vi "CRYAcquisition.vi"(0 "Setup in":T2={"No.VI"=0, "Category"="", "StepName"="", "Seq setup flattened"="", "Comment"="", "Steps config."=[], "Jump config"=[], "Start"=0.0, "Increment"=0.0, "Name"="Pa", "Unit"="Pa", "Y data"=1, "Y prefix"="", "Y dB ref"=1.0, "Y unit"="", "Repeat State Array"=[]} {"Repeat State Array"."Start" format="%#_5g"; "Y dB ref" format="%.1f"; "Y data" items=["dB", "Lin"]; "Start" format="%#_5g"}, 5 "Data In":T1[](array[typedef]) {"Z data" items=["dB", "Lin"]; "X data" items=["dB", "Lin"]; "Y data" items=["dB", "Lin"]; "Z dB ref" format="%.1f"; "Z axis" items=["Log", "Lin"]; "X dB ref" format="%.1f"; "X axis" items=["Log", "Lin"]; "Y axis" items=["Log", "Lin"]; "Y dB ref" format="%.1f"; "Curve"."z" format="%.2f"; "Curve"."y" format="%.2f"; "Curve"."x" format="%.2f"}, 7 "Results In":T4 {"Margin" format="%.2f"}, 9 "Seq Setup in":string, 11 "Step name":string="Play & Record", 12 "Hardware in":string, 13 "Calibration in":string) -> (3 "Types Out":string[](array[string]), 4 "Inserted Names Out":string[](array[string]), 6 "Data out":T1[](array[typedef]) {"Z data" items=["dB", "Lin"]; "X data" items=["dB", "Lin"]; "Y data" items=["dB", "Lin"]; "Z dB ref" format="%.1f"; "Z axis" items=["Log", "Lin"]; "X dB ref" format="%.1f"; "X axis" items=["Log", "Lin"]; "Y axis" items=["Log", "Lin"]; "Y dB ref" format="%.1f"; "Curve"."z" format="%.2f"; "Curve"."y" format="%.2f"; "Curve"."x" format="%.2f"}, 8 "Results out":T4 {"Margin" format="%.2f"}, 10 "Wave out":T3[](array[typedef]) {"Y dB ref" format="%.1f"; "Y axis" items=["Log", "Lin"]; "Y data" items=["dB", "Lin"]; "X data" items=["dB", "Lin"]})   [LabVIEW 2013]
doc: "This VI uses the Windows '95 multimedia system to play an audio waveform stream, and simultaneously record an input stream."
uses:
  Typedef Control/CRYResult Cluster Array.ctl
  Typedef Control/CRYResult Cluster.ctl
  Typedef Control/CRYData Cluster.ctl
  Typedef Control/CRYWaveform Cluster.ctl
  Typedef Control/CRYStep.ctl
  CRYMainGlobal.vi
  Misc/CRYOptions.vi
  Misc/SubVI/CRYMisc vis settings global.vi
  Calibration/SubVI/CRYCal Global.vi
  Task Sequence/CRYProject Run Control Global.vi
  CRYSound.dll
  Hardware/SubVI/CRY6175APT_Win32.dll
panel:
  in  "Record [ms]":dbl
  out "Acquisition Type":u16
  out "Index for testinfor":i32
  out "Numeric":i32
  in  "Datum":T1={"Name"="", "Curve"=[], "X data"=1, "Y data"=1, "Z data"=1, "X axis"=0, "Y axis"=1, "Z axis"=1, "X unit"="", "Y unit"="", "Z unit"="", "X dB ref"=1.0, "Y dB ref"=1.0, "Z dB ref"=1.0, "single val"=FALSE, "protected"=FALSE, "display X"=TRUE, "display Y"=FALSE, "display Z"=TRUE, "Test Info"="", "Step No."=0, "Plot Settings"={"Color"=0, "Interpolation"=0, "Point Style"=0, "Line Style"=0, "Point Color"=0, "Line Width"=0, "Bar Plot Style"=0, "Fill To"=0}, "AutoProtect"=FALSE} {"Z data" items=["dB", "Lin"]; "X data" items=["dB", "Lin"]; "Y data" items=["dB", "Lin"]; "Z dB ref" format="%.1f"; "Z axis" items=["Log", "Lin"]; "X dB ref" format="%.1f"; "X axis" items=["Log", "Lin"]; "Y axis" items=["Log", "Lin"]; "Y dB ref" format="%.1f"; "Curve"."z" format="%.2f"; "Curve"."y" format="%.2f"; "Curve"."x" format="%.2f"}
  out "Verdict":bool=TRUE
  out "Y dB ref":dbl
  in  "Waveform Cluster":T3={"Waveform"={"X0"=0.0, "dX"=0.0, "Y"=[]}, "X data"=1, "Y data"=1, "Y axis"=1, "X unit"="s", "Y unit"="V", "Y dB ref"=1.0, "display Y"=TRUE, "display X"=TRUE, "Overload?"=FALSE, "Test Info"="", "Step No."=0, "Name"="", "protected"=FALSE, "Sqc history"=[], "Signal Channel ID"=0, "Plot Settings"={"Color"=0, "Interpolation"=0, "Point Style"=0, "Line Style"=0, "Point Color"=0, "Line Width"=0, "Bar Plot Style"=0, "Fill To"=0}, "AutoProtect"=FALSE} {"Y dB ref" format="%.1f"; "Y axis" items=["Log", "Lin"]; "Y data" items=["dB", "Lin"]; "X data" items=["dB", "Lin"]}
  in  "ntaskID":u32
  in  "interact rec":bool
  in  "Record Delay":dbl caption="ms" format="%.1f"
  in  "interact play":bool
  in  "Max Out":dbl=3.0 format="%.3f"
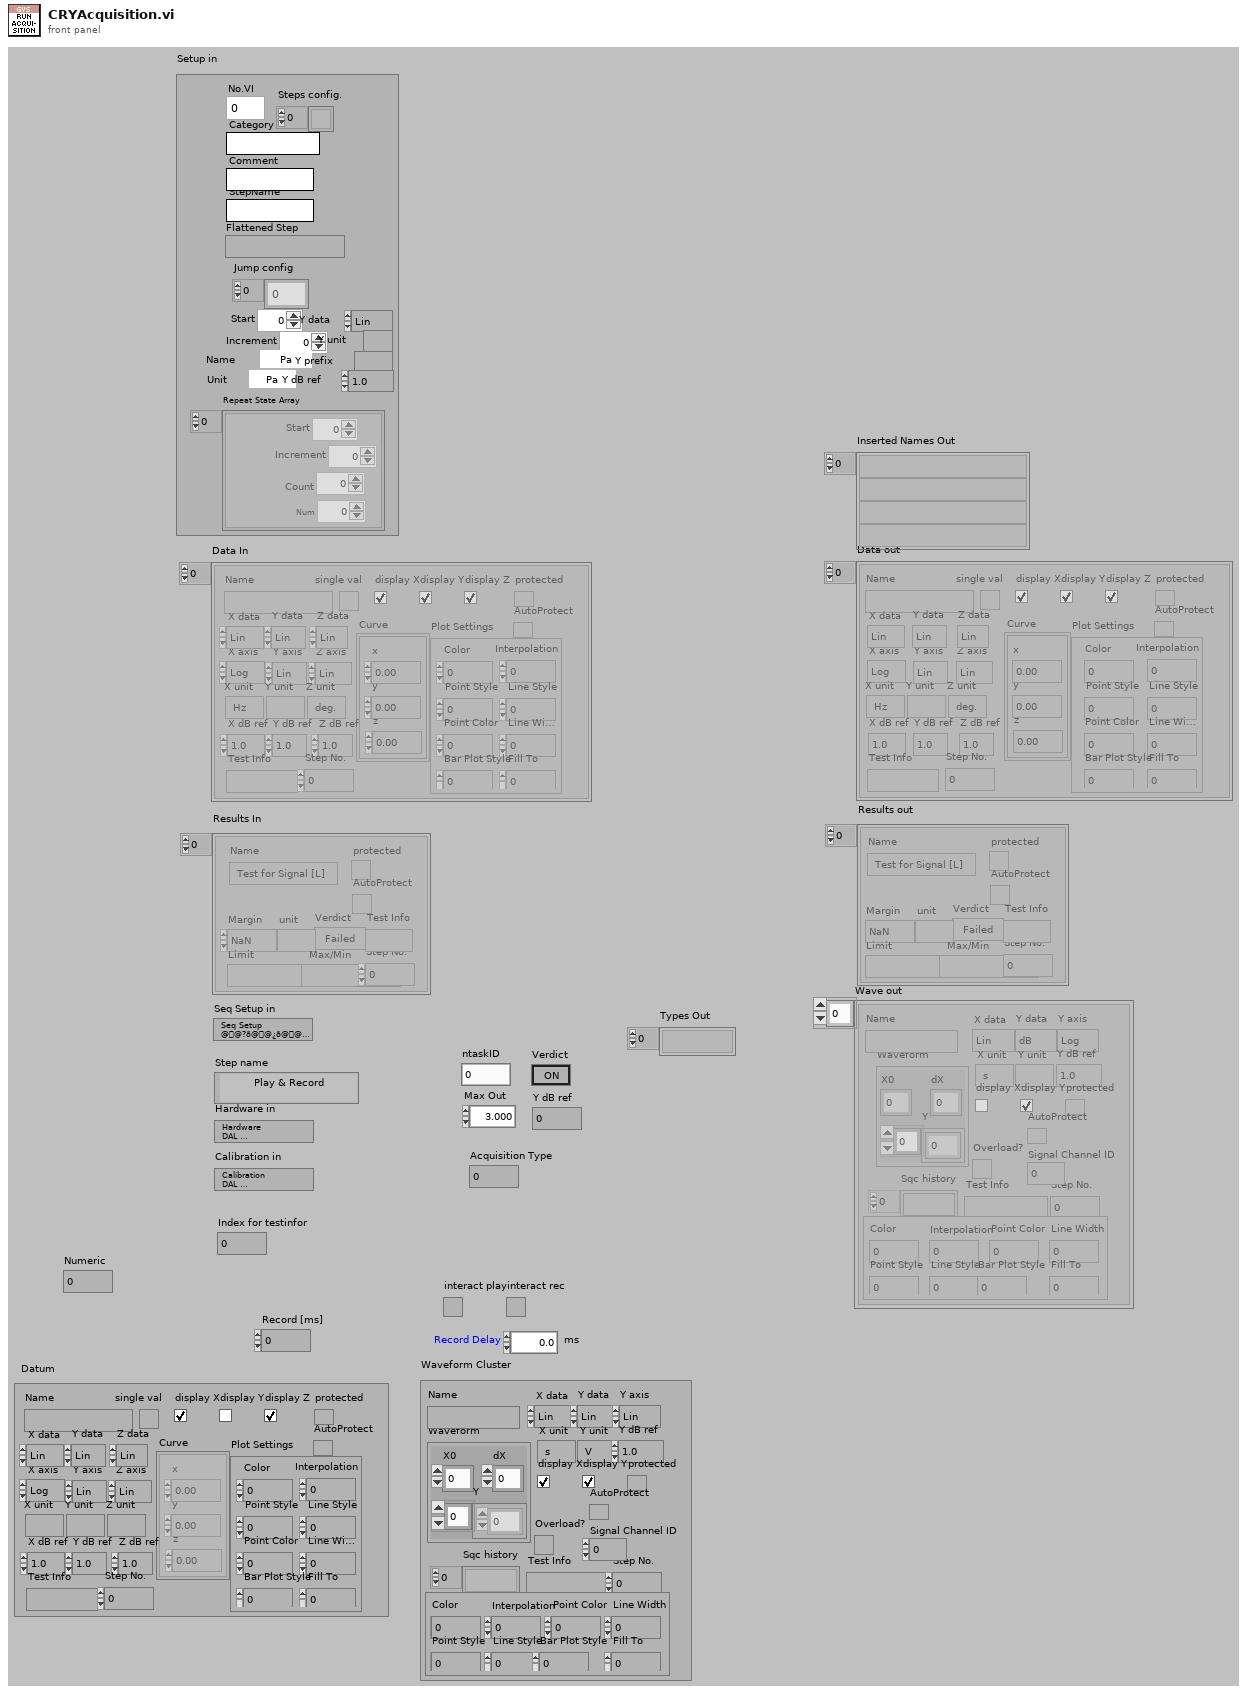
[diagram p1: front panel]
types:
  T1 = typedef "CRYData Cluster.ctl" = cluster{"Name":string, "Curve":cluster{"x":dbl, "y":dbl, "z":dbl}[], "X data":u16, "Y data":u16, "Z data":u16, "X axis":u16, "Y axis":u16, "Z axis":u16, "X unit":string, "Y unit":string, "Z unit":string, "X dB ref":dbl, "Y dB ref":dbl, "Z dB ref":dbl, "single val":bool, "protected":bool, "display X":bool, "display Y":bool, "display Z":bool, "Test Info":string, "Step No.":i32, "Plot Settings":cluster{"Color":u32, "Interpolation":u8, "Point Style":u8, "Line Style":u8, "Point Color":u32, "Line Width":u8, "Bar Plot Style":u8, "Fill To":i16}, "AutoProtect":bool}
  T2 = typedef "CRYStep.ctl" = cluster{"No.VI":i32, "Category":string, "StepName":string, "Seq setup flattened":string, "Comment":string, "Steps config.":bool[], "Jump config":i32[], "Start":dbl, "Increment":dbl, "Name":string, "Unit":string, "Y data":u16, "Y prefix":string, "Y dB ref":dbl, "Y unit":string, "Repeat State Array":cluster{"Start":dbl, "Increment":dbl, "Count":i32, "Num":i32}[]}
  T3 = typedef "CRYWaveform Cluster.ctl" = cluster{"Waveform":cluster{"X0":dbl, "dX":dbl, "Y":sgl[]}, "X data":u16, "Y data":u16, "Y axis":u16, "X unit":string, "Y unit":string, "Y dB ref":dbl, "display Y":bool, "display X":bool, "Overload?":bool, "Test Info":string, "Step No.":i32, "Name":string, "protected":bool, "Sqc history":string[], "Signal Channel ID":i32, "Plot Settings":cluster{"Color":u32, "Interpolation":u8, "Point Style":u8, "Line Style":u8, "Point Color":u32, "Line Width":u8, "Bar Plot Style":u8, "Fill To":i16}, "AutoProtect":bool}
  T4 = typedef "CRYResult Cluster Array.ctl" = T5[]
  T5 = typedef "CRYResult Cluster.ctl" = cluster{"Name":string, "Margin":dbl, "unit":string, "Verdict":bool, "Limit":string, "Max/Min":string, "protected":bool, "Step No.":i32, "Test Info":string, "AutoProtect":bool}
  T6 = enum16{"OK", "Yes", "YesNo", "YesNoCancel", "ReplaceAppend"}
  T7 = enum16{"Play & Record", "Record", "Sine Generator", "Voltmeter", "Oscilloscope", "Spectrum Analyzer", "RTA", "Generator & Voltmeter", "Generator & Oscilloscope", "Generator & Spectrum", "Generator & RTA"}
  T8 = typedef "CRYAcquisition Cluster.ctl" = cluster{"Mode":u16, "Name":string, "use ch name":bool, "Record Time":dbl, "hide rec":bool, "hide play":bool, "rec delay":dbl, "rec pad":dbl, "dcc units":i8, "sine gen setting":string, "scope_fft setting":string, "voltmeter setting":string, "rta setting":string, "trig offset(sec)":dbl, "triggered  record":bool, "trig level":dbl, "trig unit":u8, "trig slop":bool, "trig timeout(sec)":dbl, "add record":bool, "EQ":bool, "record table":string[][], "play table":string[][], "trig channel":string, "Help":string}
  T9 = typedef "CRYCalibration 2DCluster.ctl" = cluster{"Calibration":T10, "Corr Curve":T1, "EQ Curve":T1, "Sens Curve":T1}
  T10 = typedef "CRYCalibration Cluster.ctl" = cluster{"Calibration Step Name":string, "Device":string, "Correction Curve Name":string, "Equalization Curve Name":string, "Sensitivity Curve Name":string, "Corr Folder and File":string, "EQ Folder and File":string, "Sens Folder and File":string, "Corr Step size":u16, "EQ Step size":u16, "Input":bool, "Last Cal Date (sec)":timestamp, "Cha Name":string, "Corr Curve Found":bool, "EQ Curve Found":bool, "Sens Curve Found":bool, "Signal Type":string, "Calibrated Device":string, "Hz":u32}
  T11 = typedef "CRYCalibration All Cluster.ctl" = cluster{"Calibration 2D":T9[], "Help":string, "Tab Value":i32, "Input Signal Type":string, "Output Signal Type":string}
  T12 = typedef "CRYHardware Channel Info.ctl" = cluster{"ID":i32, "Name":string, "Digital":bool, "Input":bool, "Device Name":string, "Hardware Ch ID":u8, "Vmax (V)":dbl, "Latency (samples)":dbl, "Sampling Rate (Hz)":u32, "Bit Depth":u32, "Anti-aliasing Factor (%fs)":sgl, "DAQmx Channel":tag, "term config":i32, "Coupling":i32, "IEPE en":bool, "ASIOChannel Name":string, "Audio Driver":u16, "ASIOChannel Index":u8}
  T13 = typedef "CRYWaveform Cluster Array.ctl" = T3[]
  T14 = typedef "CRYData Cluster Array.ctl" = T1[]
  T15 = cluster{"MME Record Cluster":cluster{"RecDeviceID":u32, "RecSampleFreq":u32, "RecChannels":u32, "RecBitDepth":u32, "RecSampleData":i32[], "RecDataLength":u32, "RecTime":sgl, "RecLatency":sgl, "RecPadding":sgl, "nBufferUse":u32, "nRealTime":u32, "Anti Alias":u32, "Device Name":string, "Audio Driver":u16}[], "ASIO Record Cluster":cluster{"RecDeviceID":u32, "RecSampleFreq":u32, "RecChannels":u32, "RecBitDepth":u32, "RecSampleData":i32[], "RecDataLength":u32, "RecTime":sgl, "RecLatency":sgl, "RecPadding":sgl, "nBufferUse":u32, "nRealTime":u32, "Anti Alias":u32, "Device Name":string, "Audio Driver":u16}[]}
  T16 = cluster{"MME Play Cluster":cluster{"InSampleFreq":u32, "nInBitDepth":u32, "nInChannels":u32, "InSignalData":sgl[], "InSampleLen":u32, "PlayDeviceID":u32, "PlaySampleFreq":u32, "PlayChannels":u32, "PlayBitDepth":u32, "PlayMode":u32, "PlayDuration":sgl, "PlaynTimes":u32, "PlayOutLevel":sgl, "Device Name":string}[], "ASIO Play Cluster":cluster{"InSampleFreq":u32, "nInBitDepth":u32, "nInChannels":u32, "InSignalData":sgl[], "InSampleLen":u32, "PlayDeviceID":u32, "PlaySampleFreq":u32, "PlayChannels":u32, "PlayBitDepth":u32, "PlayMode":u32, "PlayDuration":sgl, "PlaynTimes":u32, "PlayOutLevel":sgl, "Device Name":string}[]}
  T17 = cluster{"RecDeviceID":u32, "RecSampleFreq":u32, "RecChannels":u32, "RecBitDepth":u32, "RecSampleData":i32[], "RecDataLength":u32, "RecTime":sgl, "RecLatency":sgl, "RecPadding":sgl, "nBufferUse":u32, "nRealTime":u32, "Anti Alias":u32, "Device Name":string, "Audio Driver":u16}[]
  T18 = cluster{"InSampleFreq":u32, "nInBitDepth":u32, "nInChannels":u32, "InSignalData":sgl[], "InSampleLen":u32, "PlayDeviceID":u32, "PlaySampleFreq":u32, "PlayChannels":u32, "PlayBitDepth":u32, "PlayMode":u32, "PlayDuration":sgl, "PlaynTimes":u32, "PlayOutLevel":sgl, "Device Name":string}[]
  T19 = typedef "CRYStimulus Test Infor Cluster.ctl" = cluster{"Stimulus Type":string, "Signal Type":string, "In/Out":bool, "FAPS":cluster{"freq":dbl, "ampl":dbl, "cycles":dbl, "samples":i32}[], "Sampling Rate":dbl, "Samples":i32, "Analysis Param":string, "Resolution":u16, "Steps":u32, "Analysis Value":dbl[], "Diff Freq":dbl, "FStart":dbl, "FStop":dbl, "Calibration Param":string, "Anti Alias":dbl, "Level Out1":dbl, "Level Out2":dbl, "EQ":bool}
  T20 = cluster{"gen'r mode":i32, "frequency":u32, "output level":dbl, "wave path":string, "wav play mode":i32, "duration":dbl, "n times":i32, "channel":i32, "wav level":dbl, "EQ":bool, "f knob log":bool, "f knob low":dbl, "f knob high":dbl, "ol knob log":bool, "ol knob low":dbl, "ol knob high":dbl, "Lin Display Prefs":string, "dB Display Prefs":string, "Duration noise":dbl, "Min freq noise":dbl, "Max freq noise":dbl, "Channel String":string, "Play Sine Wave":i32}
  T21 = typedef "CRYMultimeter.ctl" = cluster{"Ave/Max/Min":i32, "Level":i32, "Channel":i32, "Signal Type":string, "Weighting":string, "Applay Correction":bool, "lin/exp avg":u16, "rec time (sec)":dbl, "Average Time (Sec)":dbl, "Lin Display Prefs":string, "dB Display Prefs":string, "Time Weighting":u16, "Display":u16}
  T22 = cluster{"InputLevel":dbl, "unit":string, "dB ref.":dbl}
  T23 = cluster{"Bundle Element":dbl, "InputLevel":dbl, "Bundle Element":dbl}
  T24 = cluster{"Bundle Element":dbl, "InputLevel":dbl, "Bundle Element":dbl}[]
  T25 = typedef "CRYScope-FFT.ctl" = cluster{"window":i32, "n avgs":i32, "lin/exp avg":i32, "pwr/cplx avg":i32, "time (ms)":dbl, "fft lines":i32, "scope/fft mode":i32, "channel":i32, "trig. channel":i32, "Applay Correction":bool, "Time Display":string, "Freq. Weighting":string, "Ave/Max/Min":u16, "Trigger Level":dbl, "Trigger Unit":u16, "Trigger Time Offset":dbl, "Trigger Slope":u16, "Trigger/Free Run":bool, "continuous":bool, "Spectrum Display":string, "Calc FFT":bool, "Y-axis":string, "Signal Type":string}
  T26 = cluster{"Fs":dbl, "df":dbl, "db ref":dbl, "X data":u16, "Y axis":u16, "Y Unit":string, "Y":dbl[], "Max Level":dbl}
  T27 = cluster{"octave":i32, "det time":i32, "det sec":dbl, "lin/exp":i32, "weighting":i32, "channel":i32, "Ave/Max/Min":u16, "continuous":bool, "Applay Correction":bool, "Display":u16, "Channel String":string}
  T28 = cluster{"Fs":dbl, "df":dbl, "db ref":dbl, "X data":u16, "Y data":u16, "Y Unit":string}
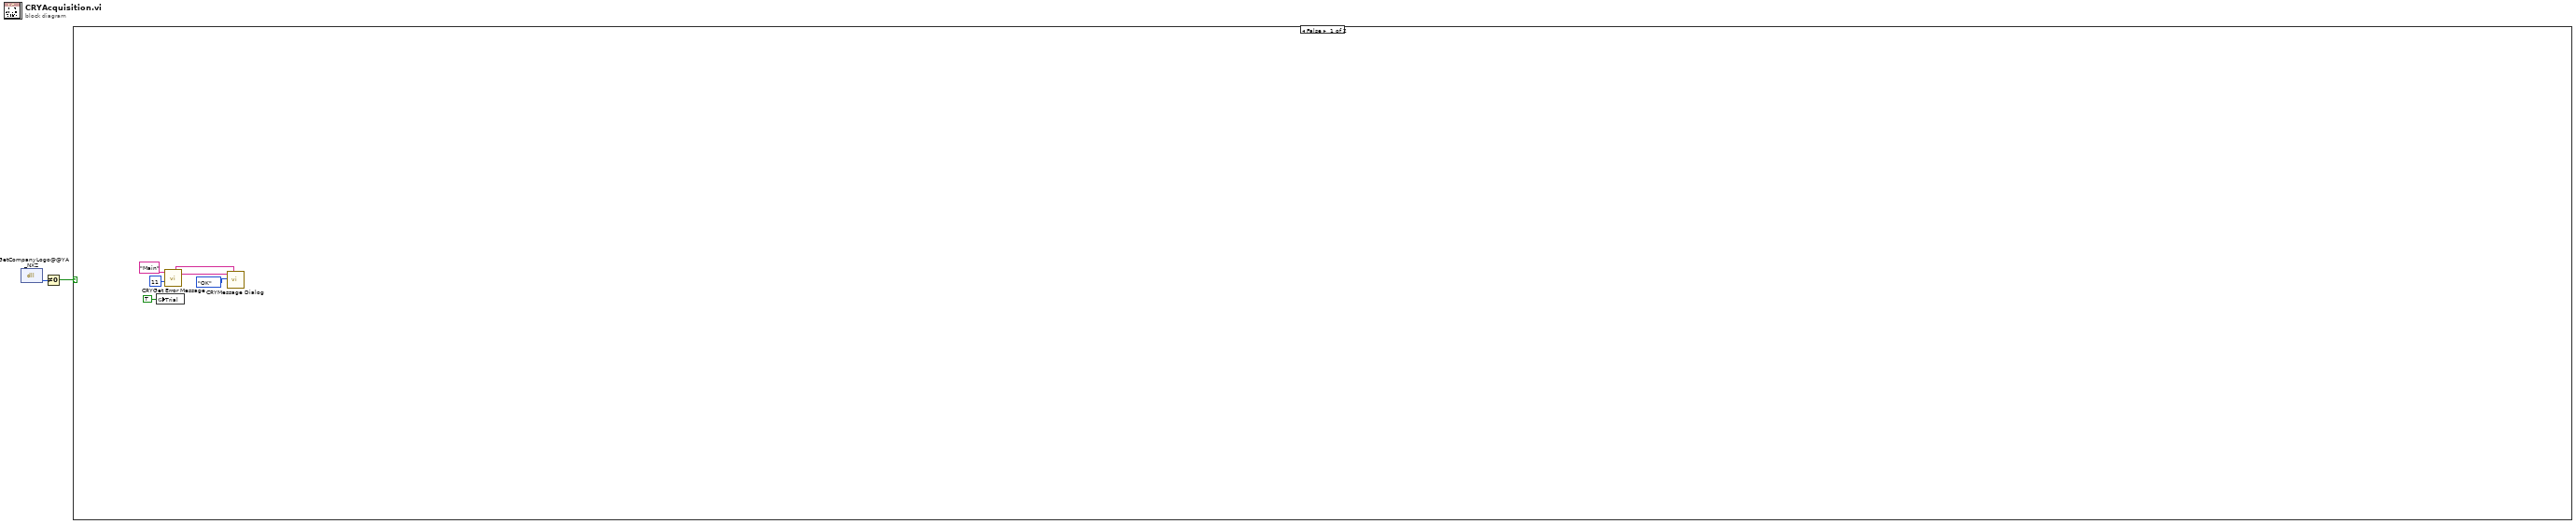
[diagram p0: block diagram]
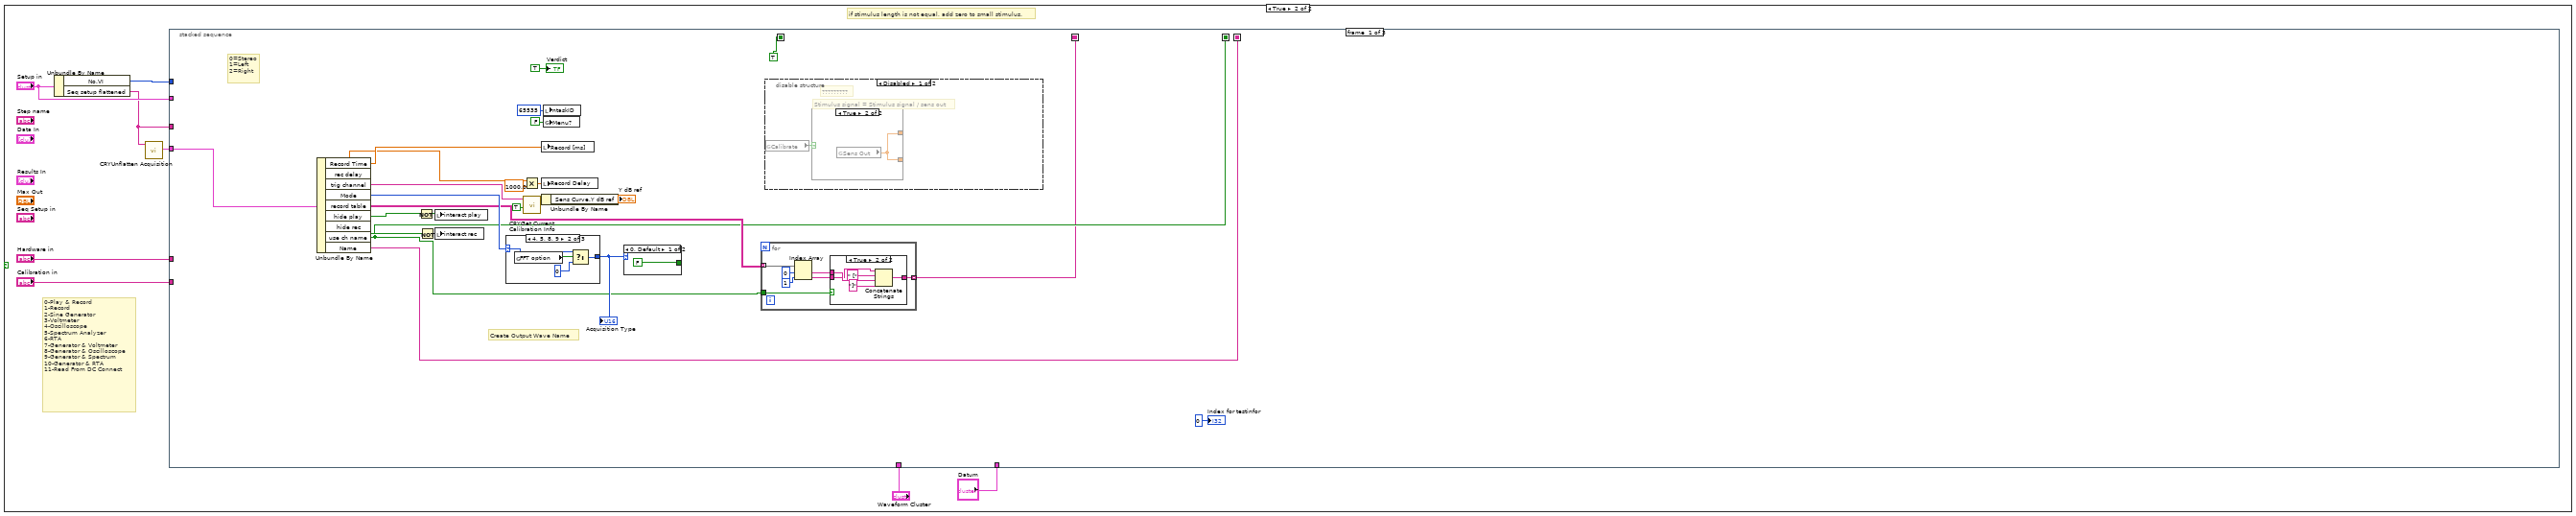
[diagram p2: hidden frame]
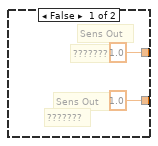
[diagram p4: hidden frame]
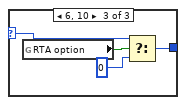
[diagram p7: hidden frame]
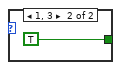
[diagram p8: hidden frame]
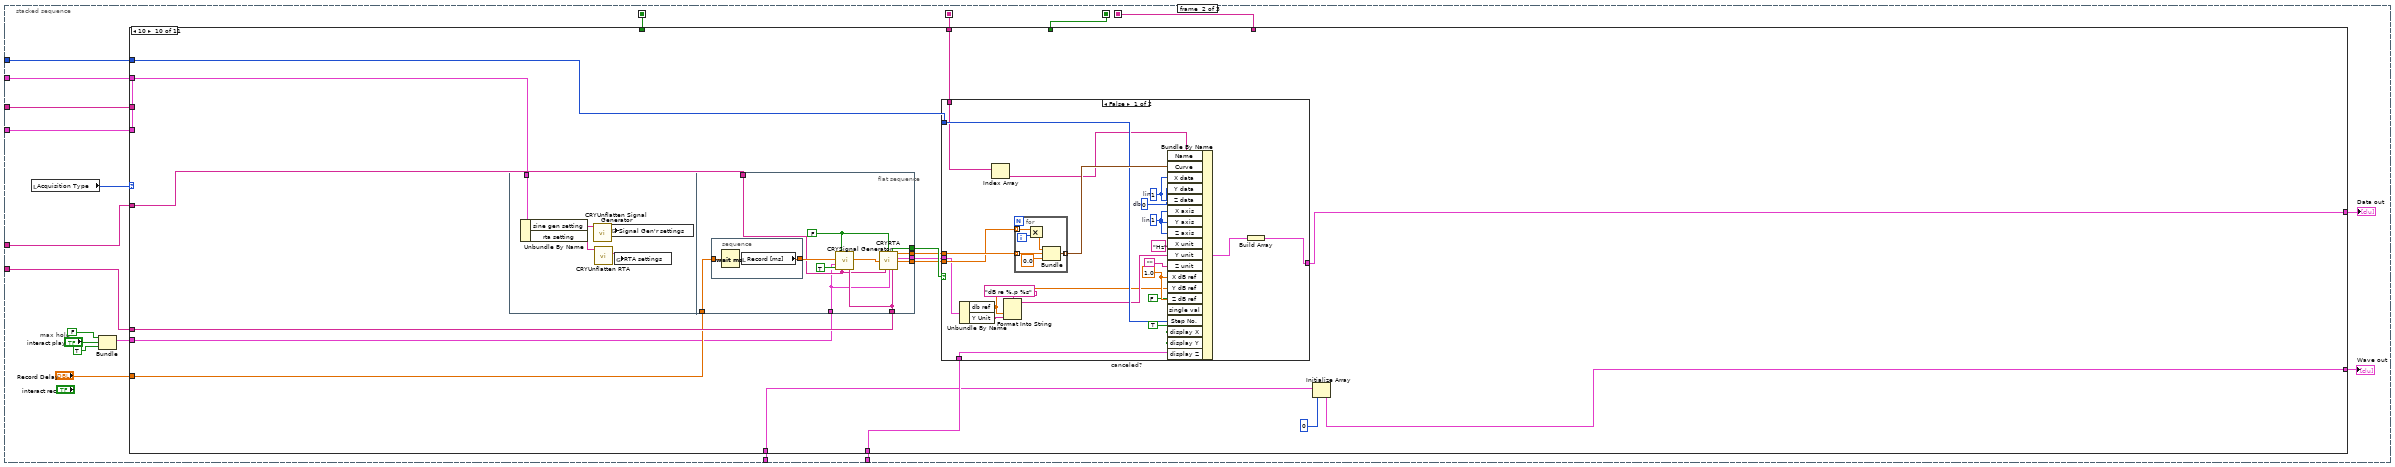
[diagram p9: hidden frame]
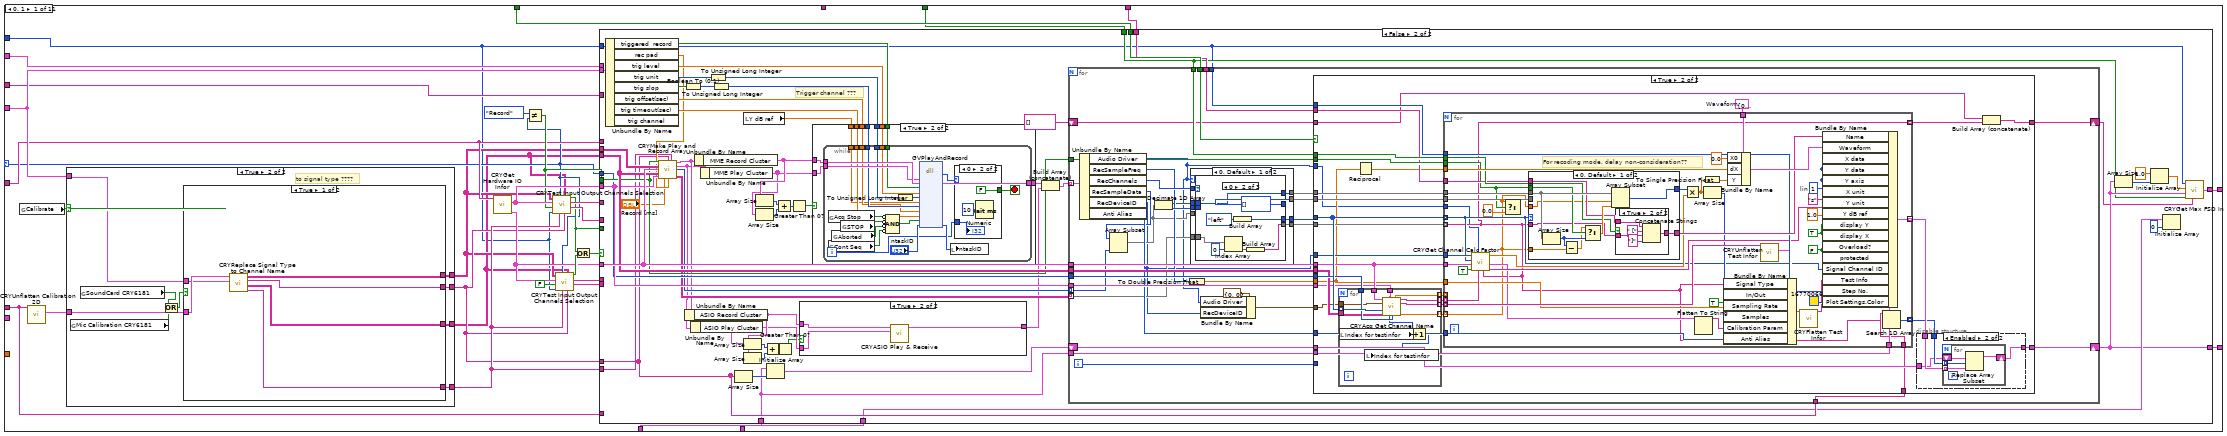
[diagram p10: hidden frame]
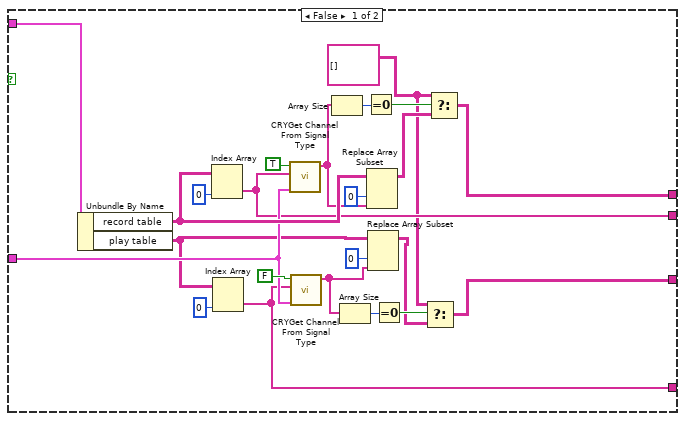
[diagram p11: hidden frame]
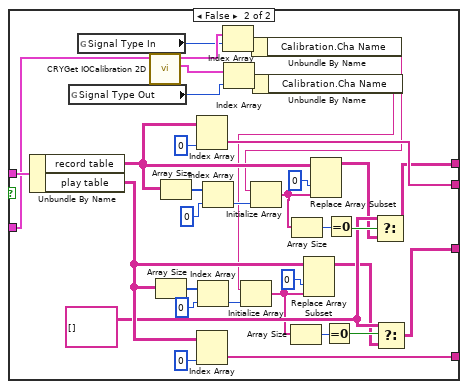
[diagram p12: hidden frame]
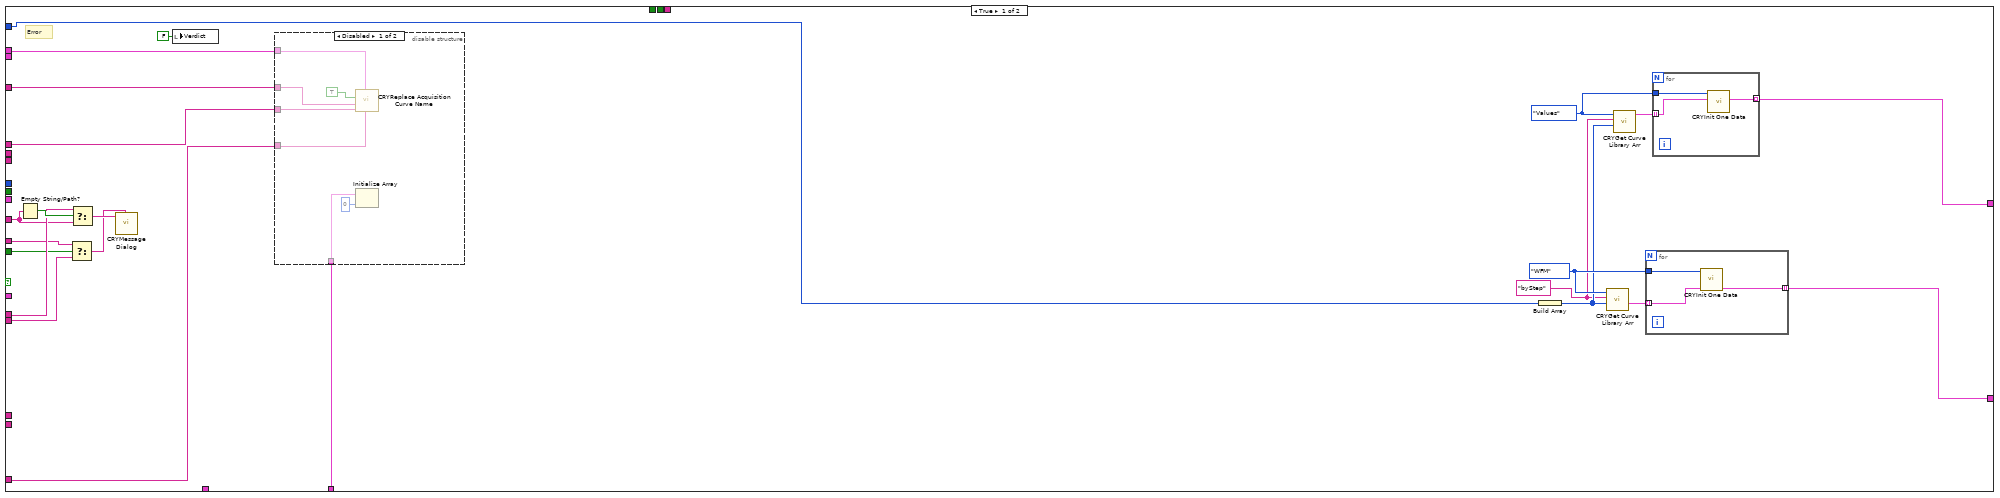
[diagram p13: hidden frame]
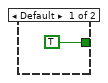
[diagram p17: hidden frame]
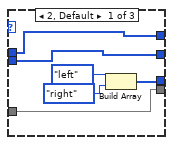
[diagram p18: hidden frame]
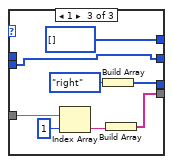
[diagram p19: hidden frame]
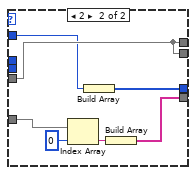
[diagram p20: hidden frame]
diagram:
  n1 = dll-call lib="D:/A_CRYSoundLab_Work/CRY6181/CRYSystem/Hardware/SubVI/CRY6175APT_Win32.dll" fn="?GetCompanyLogo@@YA_NXZ"() -> ("return type"=w2:i32)  [unwired: 3 in, 2 out]
  n2 = Not Equal To 0?(x=w2) -> (x != 0?=w1:bool)
  n3 = case shown="False" w1 {
    frame False {
      n4 = global write "CRYMainGlobal.vi" "Trial"(TRUE ("Trial")) -> ()
      n5 = call "CRYGet Error Message.vi"("Error No"=11, "Kind"="Main") -> ("Message"=w8:string, "Window Title"=w4:string)  [unwired: 4 in, 4 out]
      n6 = call "CRYMessage Dialog.vi"("Window Title"=w4, "YesNoCancel"=T6."OK", "Message Content"=w8) -> ()  [unwired: 7 in, 2 out]
    }
    frame True {
      # "0-Play & Record\n1-Record\n2-Sine Generator\n3-Voltmeter\n4-Oscilloscope\n5-Spectrum Analyzer\n6-RTA\n7-Generator & Voltmeter\n8-Generator & Oscilloscope\n9-Generator & Spectrum\n10-Generator & RTA\n11-Read From DC Connect"
      # "if stimulus length is not equal, add zero to small stimulus."
      n7 = Unbundle By Name("Setup in") -> ("No.VI"=w15:i32, "Seq setup flattened"=w11:string)
      n8 = call "CRYUnflatten Acquisition.vi"("Flatten Acquisition"=w11) -> ("Acquisition"=w9:T8)  [unwired: 10 out]
      n9 = stacked-sequence {
        seq-local: [TRUE ("add record") _ _] -> [_ w87 _]
        seq-local: [w19 _ _] -> [_ w80 _]
        seq-local: [w18 _ _] -> [_ w79 _]
        seq-local: [w20 _ _] -> [_ w78 _]
        tunnel: "Datum" -> [_ w88 _]
        tunnel: "Waveform Cluster" -> [_ w81 _]
        tunnel: w11 -> [_ w75 _]
        tunnel: w15 -> [_ w77 w1061]
        tunnel: "Setup in" -> [_ w76 w1065]
        tunnel: "Calibration in" -> [_ w74 _]
        tunnel: "Hardware in" -> [_ w73 _]
        tunnel: w9 -> [w26 w72 _]
        frame #0 {
          # "Create Output Wave Name"
          # "0=Stereo\n1=Left\n2=Right"
          n10 = Unbundle By Name(w26) -> ("Record Time"=w37:dbl, "rec delay"=w35:dbl, "trig channel"=w25:string, "Mode"=w24:u16, "record table"=w21:string[][], "hide play"=w23:bool, "hide rec"=w22:bool, "use ch name"=w20:bool, "Name"=w18:string)
          n11 = Not(x=w23) -> (.not. x?=w40:bool)
          n12 = Not(x=w22) -> (.not. x?=w39:bool)
          n13 = local write "interact play"(w40) -> ()
          n14 = local write "interact rec"(w39) -> ()
          n15 = case shown="4, 5, 8, 9" w24 {
            selector: w24 -> [w58 w59 w63]
            tunnel: [w58 w61 w65] -> w38
            frame Default {
            }
            frame 4, 5, 8, 9 {
              n16 = global read "CRYOptions.vi" "FFT option"() -> (w62:bool)
              n17 = Select(t=w59, s=w62, f=u16 0) -> (s? t:f=w61:u16)
            }
            frame 6, 10 {
              n18 = global read "CRYOptions.vi" "RTA option"() -> (w66:bool)
              n19 = Select(t=w63, s=w66, f=u16 0) -> (s? t:f=w65:u16)
            }
          }
          "Acquisition Type" <- w38
          n20 = Multiply(x=w35, y=1000.0) -> (x*y=w36:dbl)
          n21 = call "CRYGet Current Calibration Info.vi"("Is Input?"=TRUE, "Signal Type Name"=w25) -> ("Calibration All Cluster"=w31:T9)  [unwired: 9 in]
          n22 = local write "Record [ms]"(w37) -> ()
          n23 = local write "Record Delay"(w36) -> ()
          n24 = Unbundle By Name(w31) -> ("Sens Curve.Y dB ref"=→"Y dB ref":dbl)
          n25 = local write "ntaskID"(u32 65535 ("ntaskID")) -> ()
          n26 = global write "CRYMisc vis settings global.vi" "Menu?"(FALSE ("Menu?")) -> ()
          n27 = case shown="0, Default" w38 {
            tunnel: [FALSE TRUE] -> _
            frame 0, Default {
            }
            frame 1, 3 {
            }
          }
          n28 = for {
            tunnel: w21 -> [w45] mode=indexing
            tunnel: w20 -> [w44]
            tunnel: [w41] -> w19 mode=indexing
            n29 = Index Array(array=w45, index #1=0 ("index"), index #2=1 ("index")) -> (element #1=w43:string, element #2=w42:string)
            n30 = case shown="True" w44 {
              tunnel: w43 -> [_ w51]
              tunnel: [w48 w50] -> w41
              tunnel: w42 -> [w48 w49]
              frame False {
              }
              frame True {
                n31 = Concatenate Strings(w49, " [" ("string"), w51, "]" ("string")) -> (w50:string)
              }
            }
          }
          n32 = disable-structure shown="Disabled" {
            frame Disabled {
              # "?????????"
              # "Stimulus signal = Stimulus signal / sens out"
              n33 = global read "CRYCal Global.vi" "Calibrate"() -> (w54:bool)
              n34 = case shown="True" w54 {
                tunnel: [1.0 ("Sens Out") w57] -> _
                tunnel: [1.0 ("Sens Out") w57] -> _
                frame False {
                  # "???????"
                  # "???????"
                  # "Sens Out"
                  # "Sens Out"
                }
                frame True {
                  n35 = global read "CRYCal Global.vi" "Sens Out"() -> (w57:dbl)
                }
              }
            }
            frame Enabled {
            }
          }
          "Verdict" <- TRUE ("Verdict")
          "Index for testinfor" <- 0 ("Index Play")
        }
        frame #1 {
          # "max hold"
          n36 = local read "Acquisition Type"() -> (w69:u16)
          n37 = Bundle(FALSE, "interact play"="interact play", TRUE) -> (w86:cluster{bool, "interact play":bool, bool})  [unwired: 1 out]
          n38 = case shown="10" w69 {
            selector: w69 -> [w92 _ _ _ _ _ _ _ _ _ _]
            tunnel: w73 -> [w100 w541 w562 w611 w671 w731 w783 w841 w909 w972 _]
            tunnel: w74 -> [w94 w540 w561 w610 w670 w730 w784 w840 w908 w977 _]
            tunnel: [w120 w543 w565 w599 w669 w727 w788 w827 w905 w976 w1049] -> w71
            tunnel: w88 -> [w119 w544 w566 w600 w660 w729 w787 w828 w906 w975 w1048]
            tunnel: w87 -> [w118 _ _ _ _ _ _ _ _ _ _]
            tunnel: w86 -> [_ w539 w559 w608 w666 w725 w780 w837 w902 w970 _]
            tunnel: "Record Delay" -> [_ _ _ _ _ _ w781 w838 w904 w973 _]
            tunnel: w72 -> [w104 w542 w560 w609 w667 w726 w782 w839 w903 w971 _]
            tunnel: w81 -> [w110 w537 w557 w607 w664 w723 w778 w835 w900 w968 w1052]
            tunnel: [w109 w536 w556 w606 w663 w722 w777 w834 w899 w967 w1051] -> w70
            tunnel: w80 -> [_ _ w554 w601 w659 w721 w776 w833 w898 w966 w1028]
            tunnel: w79 -> [w108 _ _ _ _ _ _ _ _ _ _]
            tunnel: w77 -> [w89 _ w555 w603 w661 w718 w775 w831 w896 w963 w1047]
            tunnel: w78 -> [w106 _ _ w598 _ _ _ w829 _ _ _]
            tunnel: w76 -> [w99 _ _ _ _ _ _ _ _ _ _]
            tunnel: w75 -> [w98 _ _ _ _ _ _ _ _ _ _]
            frame 0, 1 {
              n39 = global read "CRYCal Global.vi" "Calibrate"() -> (w107:bool)
              n40 = call "CRYUnflatten Calibration 2D.vi"("Flattened Calibration"=w94) -> ("Calibration Step Out"=w97:T11)  [unwired: 8 in, 2 out]
              n41 = case shown="True" w107 {
                tunnel: [w127 w147] -> w91
                tunnel: [w121 w148] -> w90
                tunnel: w104 -> [w143 w152]
                tunnel: w97 -> [w135 w149]
                tunnel: [w133 w151] -> w95
                tunnel: [w132 w150] -> w93
                frame False {
                  w122 = string[][] [] ("output array")
                  n42 = Unbundle By Name(w143) -> ("record table"=w140:string[][], "play table"=w134:string[][])
                  n43 = Index Array(array=w140, index (col)=0 ("disabled index (col)")) -> (element=w132:string[])  [unwired: 1 in]
                  n44 = Index Array(array=w134, index (col)=0 ("disabled index (col)")) -> (element=w133:string[])  [unwired: 1 in]
                  n45 = call "CRYGet Channel From Signal Type.vi"("Calibration"=w135, "Signal Type Name Array In"=w132, "In/Out?"=TRUE) -> ("Channel Name Array Out"=w131:string[])  [unwired: 7 in, 1 out]
                  n46 = call "CRYGet Channel From Signal Type.vi"("Calibration"=w135, "Signal Type Name Array In"=w133, "In/Out?"=FALSE) -> ("Channel Name Array Out"=w125:string[])  [unwired: 7 in, 1 out]
                  n47 = Array Size(array=w131) -> (size(s)=w130:i32)
                  n48 = Array Size(array=w125) -> (size(s)=w126:i32)
                  n49 = Equal To 0?(x=w130) -> (x = 0?=w129:bool)
                  n50 = Replace Array Subset(array=w140, new element=w131, index (col)=0 ("disabled index (col)")) -> (w128:string[][])  [unwired: 1 in]
                  n51 = Replace Array Subset(array=w134, new element=w125, index (col)=0 ("disabled index (col)")) -> (w123:string[][])  [unwired: 1 in]
                  n52 = Equal To 0?(x=w126) -> (x = 0?=w124:bool)
                  n53 = Select(t=w122, s=w124, f=w123) -> (s? t:f=w121:string[][])
                  n54 = Select(t=w122, s=w129, f=w128) -> (s? t:f=w127:string[][])
                }
                frame True {
                  # "to signal type ????"
                  n55 = global read "CRYCal Global.vi" "Mic Calibration CRY6181"() -> (w145:bool)
                  n56 = global read "CRYCal Global.vi" "SoundCard CRY6181"() -> (w146:bool)
                  n57 = Or(x=w146, y=w145) -> (x .or. y?=w144:bool)
                  n58 = case shown="True" w144 {
                    tunnel: w152 -> [w157 w190]
                    tunnel: [w153 w182] -> w151
                    tunnel: [w155 w179] -> w150
                    tunnel: w149 -> [w158 w178]
                    tunnel: [w154 w162] -> w148
                    tunnel: [w156 w159] -> w147
                    frame True {
                      n59 = call "CRYReplace Signal Type to Channel Name.vi"("Acquisition step in"=w157, "Calibration Step in"=w158) -> ("Play Signal Type"=w153:string[], "Play table"=w154:string[][], "Record Signal Type"=w155:string[], "record table"=w156:string[][])  [unwired: 6 in]
                    }
                    frame False {
                      w164 = string[][] [] ("output array")
                      n60 = Unbundle By Name(w190) -> ("record table"=w180:string[][], "play table"=w184:string[][])
                      n61 = global read "CRYCal Global.vi" "Signal Type Out"() -> (w170:u16)
                      n62 = global read "CRYCal Global.vi" "Signal Type In"() -> (w174:u16)
                      n63 = call "CRYGet IOCalibration 2D.vi"("Calibration"=w178) -> ("O_Calibration 2D Out"=w171:T9[], "I_Calibration 2D Out"=w175:T9[])  [unwired: 9 in]
                      n64 = Array Size(array=w184) -> (size(s)=w185:i32[])
                      n65 = Array Size(array=w180) -> (size(s)=w193:i32[])
                      n66 = Index Array(array=w180, index (col)=0 ("disabled index (col)")) -> (element=w179:string[])  [unwired: 1 in]
                      n67 = Index Array(array=w184, index (col)=0 ("disabled index (col)")) -> (element=w182:string[])  [unwired: 1 in]
                      n68 = Index Array(array=w185, index=0) -> (element=w188:i32)
                      n69 = Index Array(array=w193, index=0) -> (element=w189:i32)
                      n70 = Index Array(array=w175, index=w174) -> (element=w173:T9)
                      n71 = Index Array(array=w171, index=w170) -> (element=w172:T9)
                      n72 = Unbundle By Name(w173) -> ("Calibration.Cha Name"=w177:string)
                      n73 = Initialize Array(w177, w189) -> (w165:string[])
                      n74 = Unbundle By Name(w172) -> ("Calibration.Cha Name"=w176:string)
                      n75 = Initialize Array(w176, w188) -> (w161:string[])
                      n76 = Array Size(array=w161) -> (size(s)=w169:i32)
                      n77 = Array Size(array=w165) -> (size(s)=w167:i32)
                      n78 = Replace Array Subset(array=w184, new element=w161, index (col)=0 ("disabled index (col)")) -> (w163:string[][])  [unwired: 1 in]
                      n79 = Replace Array Subset(array=w180, new element=w165, index (col)=0 ("disabled index (col)")) -> (w160:string[][])  [unwired: 1 in]
                      n80 = Equal To 0?(x=w169) -> (x = 0?=w168:bool)
                      n81 = Equal To 0?(x=w167) -> (x = 0?=w166:bool)
                      n82 = Select(t=w164, s=w166, f=w160) -> (s? t:f=w159:string[][])
                      n83 = Select(t=w164, s=w168, f=w163) -> (s? t:f=w162:string[][])
                    }
                  }
                }
              }
              n84 = call "CRYGet Hardware IO Infor.vi"("Hardware setup In"=w100) -> ("I_channel Info Out"=w113:T12[], "O_channel Info Out"=w112:T12[])  [unwired: 9 out]
              n85 = Not Equal?(x=T7."Record" ("Record Mode"), y=w92) -> (x != y?=w105:bool)
              n86 = call "CRYTest Input Output Channels Selection.vi"("Record Signal Path In"=w93, "Output Selected Array"=w90, "Play Signal Path In"=w95, "Acquisition Type"=w92, "No.VI"=w89, "Play/Record"=w105, "Channel Info In"=w112, "Input Selected Array"=w91) -> ("Msg Title Str"=w102:string, "Message Str"=w115:string, "Error Flag"=w101:bool)  [unwired: 1 in]
              n87 = call "CRYTest Input Output Channels Selection.vi"("Record Signal Path In"=w93, "Output Selected Array"=w90, "Play Signal Path In"=w95, "Acquisition Type"=w92, "No.VI"=w89, "Play/Record"=FALSE, "Channel Info In"=w113, "Input Selected Array"=w91) -> ("Msg Title Str"=w103:string, "Message Str"=w114:string, "Error Flag"=w117:bool)  [unwired: 1 in]
              n88 = Or(x=w101, y=w117) -> (x .or. y?=w116:bool)
              n89 = case shown="False" w116 {
                tunnel: w92 -> [_ w267]
                tunnel: [w194 w248] -> w120
                tunnel: w119 -> [w216 w257]
                tunnel: w118 -> [_ w285]
                tunnel: w115 -> [w213 _]
                tunnel: w114 -> [w214 _]
                tunnel: w91 -> [_ w284]
                tunnel: w90 -> [_ w281]
                tunnel: w113 -> [_ w282]
                tunnel: w112 -> [_ w280]
                tunnel: w110 -> [_ w241]
                tunnel: [w199 w253] -> w109
                tunnel: w108 -> [_ w263]
                tunnel: w89 -> [w202 w251]
                tunnel: w106 -> [_ w252]
                tunnel: w105 -> [_ w270]
                tunnel: w104 -> [_ w279]
                tunnel: w103 -> [w209 _]
                tunnel: w102 -> [w210 _]
                tunnel: w101 -> [w211 _]
                tunnel: w100 -> [w205 _]
                tunnel: w99 -> [w206 _]
                tunnel: w98 -> [w204 _]
                tunnel: w93 -> [_ w260]
                tunnel: w95 -> [_ w264]
                tunnel: w94 -> [w203 _]
                frame True {
                  w198 = enum16{"Curves", "Values", "Results", "WFM"}."Values" ("Type In")
                  w196 = "byStep" ("sOption")
                  w200 = enum16{"Curves", "Values", "Results", "WFM"}."WFM" ("Type In")
                  # "Error"
                  n90 = Empty String/Path?(string/path=w213) -> (empty?=w215:bool)
                  n91 = Select(t=w210, s=w211, f=w209) -> (s? t:f=w208:string)
                  n92 = Select(t=w214, s=w215, f=w213) -> (s? t:f=w212:string)
                  n93 = call "CRYMessage Dialog.vi"("Window Title"=w208, "Message Content"=w212) -> ()  [unwired: 8 in, 2 out]
                  n94 = local write "Verdict"(FALSE ("Verdict")) -> ()
                  n95 = disable-structure shown="Disabled" {
                    disable-tunnel: w216 -> [w222 _]
                    disable-tunnel: w206 -> [w221 _]
                    disable-tunnel: w205 -> [w219 _]
                    disable-tunnel: w204 -> [w218 _]
                    disable-tunnel: w203 -> [w217 _]
                    frame Disabled {
                      n96 = call "CRYReplace Acquisition Curve Name.vi"("Calibration in"=w217, "Setup in"=w221, "Hardware Setup In"=w219, "Step Setup In"=w218, "No Insert CurveLib?"=TRUE) -> ()  [unwired: 4 in, 3 out]
                      n97 = Initialize Array(w222, 0 ("Dimension Size")) -> ()  [unwired: 1 out]
                    }
                    frame Enabled {
                    }
                  }
                  n98 = Build Array(w202) -> (w197:i32[])
                  n99 = call "CRYGet Curve Library Arr.vi"("Index"=w197, "sOption"=w196, "Type In"=w200) -> ("Waveforms"=w201:T13)  [unwired: 6 in, 2 out]
                  n100 = call "CRYGet Curve Library Arr.vi"("Index"=w197, "sOption"=w196, "Type In"=w198) -> ("Curves/Values"=w195:T14)  [unwired: 6 in, 2 out]
                  n101 = for {
                    tunnel: w201 -> [w228] mode=indexing
                    tunnel: w200 -> [w229]
                    tunnel: [w227] -> w199 mode=indexing
                    n102 = call "CRYInit One Data.vi"("Waveform In"=w228, "Type"=w229) -> ("Waveform Out"=w227:T3)  [unwired: 7 in, 2 out]
                  }
                  n103 = for {
                    tunnel: w195 -> [w225] mode=indexing
                    tunnel: w198 -> [w226]
                    tunnel: [w224] -> w194 mode=indexing
                    n104 = call "CRYInit One Data.vi"("Data In"=w225, "Type"=w226) -> ("Data Out"=w224:T1)  [unwired: 7 in, 2 out]
                  }
                }
                frame False {
                  # "Trigger channel ???"
                  n105 = Unbundle By Name(w279) -> ("triggered  record"=w269:bool, "rec pad"=w266:dbl, "trig level"=w278:dbl, "trig unit"=w277:u8, "trig slop"=w275:bool, "trig offset(sec)"=w272:dbl, "trig timeout(sec)"=w271:dbl)  [unwired: 1 out]
                  n106 = call "CRYMake Play and Record Array.vi"("Play&Record/Record"=w270, "Selected Record Signal Path In"=w260, "Selected Play Signal Path In"=w264, "Selected Record In"=w284, "input channel Info In"=w282, "Selected Play In"=w281, "output channel Info In"=w280, "Rec Time"="Record [ms]", "Rec Padding Time"=w266) -> ("Record Cluster Out"=w240:T15, "Play Cluster Out"=w239:T16, "Real Rec Len"=w265:i32[], "Record Name Array"=w262:string[][])  [unwired: 1 in, 2 out]
                  n107 = Boolean To (0,1)(Boolean=w275) -> (0, 1=w274:i16)
                  n108 = Unbundle By Name(w240) -> ("ASIO Record Cluster"=w235:T17)
                  n109 = Unbundle By Name(w239) -> ("ASIO Play Cluster"=w234:T18)
                  n110 = Unbundle By Name(w240) -> ("MME Record Cluster"=w243:T17)
                  n111 = Unbundle By Name(w239) -> ("MME Play Cluster"=w242:T18)
                  n112 = To Unsigned Long Integer(number=w277) -> (unsigned 32bit integer=w276:u32)
                  n113 = To Unsigned Long Integer(number=w274) -> (unsigned 32bit integer=w273:u32)
                  n114 = Array Size(array=w260) -> (size(s)=w261:i32)
                  n115 = local read "Y dB ref"() -> (w268:dbl)
                  n116 = Array Size(array=w234) -> (size(s)=w236:i32)
                  n117 = Array Size(array=w235) -> (size(s)=w238:i32)
                  n118 = Array Size(array=w243) -> (size(s)=w245:i32)
                  n119 = Array Size(array=w242) -> (size(s)=w246:i32)
                  n120 = Add(x=w236, y=w238) -> (x+y=w237:i32)
                  n121 = Initialize Array(w241, w261) -> (w259:T3[])
                  n122 = Add(x=w245, y=w246) -> (x+y=w247:i32)
                  n123 = Greater Than 0?(x=w237) -> (x > 0?=w233:bool)
                  n124 = Greater Than 0?(x=w247) -> (x > 0?=w244:bool)
                  n125 = case shown="True" w233 {
                    tunnel: w235 -> [w286 w289]
                    tunnel: w234 -> [_ w288]
                    tunnel: [w286 w287] -> w231
                    frame False {
                    }
                    frame True {
                      n126 = call "CRYASIO Play & Receive.vi"("ASIO Play Cluster In"=w288, "ASIO Record Cluster In"=w289) -> ("ASIO Record Cluster Out"=w287:T17)  [unwired: 9 in]
                    }
                  }
                  n127 = case shown="True" w244 {
                    tunnel: [w290 w300] -> w283
                    tunnel: w278 -> [_ w299]
                    tunnel: w276 -> [_ w298]
                    tunnel: w273 -> [_ w297]
                    tunnel: w272 -> [_ w296]
                    tunnel: w271 -> [_ w295]
                    tunnel: w269 -> [_ w294]
                    tunnel: w268 -> [_ w293]
                    tunnel: w243 -> [w290 w292]
                    tunnel: w242 -> [_ w291]
                    frame False {
                    }
                    frame True {
                      n128 = while {
                        tunnel: w292 -> [w321]
                        tunnel: w291 -> [w320]
                        tunnel: [w319] -> w300
                        tunnel: w299 -> [w310]
                        tunnel: w298 -> [w308]
                        tunnel: w297 -> [w307]
                        tunnel: w296 -> [w306]
                        tunnel: w295 -> [w305]
                        tunnel: w294 -> [w304]
                        tunnel: w293 -> [w303]
                        i -> [w301]
                        stop <- w317 stop-if-true
                        n129 = global read "CRYMainGlobal.vi" "Acq Stop"() -> (w316:bool)
                        n130 = global read "CRYProject Run Control Global.vi" "Cont Seq"() -> (w302:bool)
                        n131 = global read "CRYProject Run Control Global.vi" "Aborted"() -> (w313:bool)
                        n132 = global read "CRYMainGlobal.vi" "STOP"() -> (w314:bool)
                        n133 = Compound Arithmetic op=AND(invert w316, invert w314, invert w313, invert w302) -> (w312:bool)
                        n134 = To Unsigned Long Integer(number=w308) -> (unsigned 32bit integer=w309:u32)
                        n135 = dll-call lib="D:/A_CRYSoundLab_Work/CRY6181/CRYSound.dll" fn="GVPlayAndRecord"("playdata"=w320, "recorddata"=w321, "TrigFlag"=w304, "TrigLevel"=w310, "TrigUnit"=w309, "TrigdBRef"=w303, "TrigSlop"=w307, "TrigOffset"=w306, "TrigTimeOut"=w305, "startflag"=w312, "ntaskID"="ntaskID") -> ("return type"=w315:u32, "recorddata"=w319:T17, "ntaskID"=w318:u32)  [unwired: 4 in, 10 out]
                        n136 = local write "ntaskID"(w318) -> ()
                        n137 = case shown="0" w315 {
                          tunnel: [TRUE FALSE] -> w317
                          tunnel: w301 -> [_ w323]
                          frame Default {
                          }
                          frame 0 {
                            n138 = Wait (ms)(milliseconds to wait=u32 10) -> ()  [unwired: 1 out]
                            "Numeric" <- w323
                          }
                        }
                      }
                    }
                  }
                  n139 = Build Array (concatenate)(w283, w231) -> (w232:T17)
                  n140 = for {
                    tunnel: w232 -> [w360] mode=indexing
                    tunnel: w270 -> [w344]
                    tunnel: w241 -> [w358]
                    tunnel: w285 -> [w356]
                    shift-right: [w357] -> w253
                    shift-left: w259 -> [w355]
                    tunnel: w251 -> [w354]
                    tunnel: w282 -> [w349]
                    tunnel: w281 -> [w348]
                    tunnel: w280 -> [w347]
                    tunnel: w252 -> [w346]
                    tunnel: w267 -> [w345]
                    tunnel: w265 -> [w340] mode=indexing
                    tunnel: w262 -> [w338] mode=indexing
                    tunnel: w263 -> [w336]
                    tunnel: w260 -> [w334]
                    shift-right: [w326] -> w249
                    shift-left: string[] [] -> [w327]
                    i -> [w328]
                    n141 = Unbundle By Name(w360) -> ("Audio Driver"=w329:u16, "RecSampleFreq"=w343:u32, "RecChannels"=w359:u32, "RecSampleData"=w339:i32[], "RecDeviceID"=w331:u32, "Anti Alias"=w341:u32)
                    n142 = Array Subset(array=w339, length=w340) -> (w333:i32[])  [unwired: 1 in]
                    n143 = Decimate 1D Array(w333) -> (w342:i32[], w352:i32[])
                    n144 = To Double Precision Float(number=w343) -> (double precision float=w335:dbl)
                    n145 = case shown="0, Default" w329 {
                      tunnel: w359 -> [w368 w391]
                      tunnel: [w367 w397] -> w353
                      tunnel: w352 -> [w366 _]
                      tunnel: [w365 w392] -> w351
                      tunnel: [w364 w392] -> w350
                      tunnel: w342 -> [w363 _]
                      tunnel: w338 -> [w362 w396]
                      tunnel: [w361 w395] -> w337
                      tunnel: w333 -> [_ w392]
                      frame 0, Default {
                        n146 = case shown="0" w368 {
                          tunnel: [w371 w379 i32[] [] ("RecSampleData")] -> w365
                          tunnel: [w370 i32[] [] ("RecSampleData") w387] -> w364
                          tunnel: [w372 w380 w388] -> w367
                          tunnel: w363 -> [w371 w379 _]
                          tunnel: w366 -> [w370 _ w387]
                          tunnel: w362 -> [w369 w378 w386]
                          tunnel: [w369 w376 w383] -> w361
                          frame 2, Default {
                            n147 = Build Array(enum16{"left", "right"}."left", enum16{"left", "right"}."right") -> (w372:enum16{"left", "right"}[])
                          }
                          frame 0 {
                            n148 = Index Array(array=w378, index=0) -> (element=w377:string)
                            n149 = Build Array(enum16{"left", "right"}."left") -> (w380:enum16{"left", "right"}[])
                            n150 = Build Array(w377) -> (w376:string[])
                          }
                          frame 1 {
                            n151 = Index Array(array=w386, index=1) -> (element=w384:string)
                            n152 = Build Array(enum16{"left", "right"}."right") -> (w388:enum16{"left", "right"}[])
                            n153 = Build Array(w384) -> (w383:string[])
                          }
                        }
                      }
                      frame 2 {
                        n154 = Index Array(array=w396, index=0) -> (element=w394:string)
                        n155 = Build Array(w391) -> (w397:u32[])
                        n156 = Build Array(w394) -> (w395:string[])
                      }
                    }
                    n157 = Bundle By Name(cluster=cluster{"RecDeviceID":u32, "Audio Driver":u32} {"RecDeviceID"=0, "Audio Driver"=0} ("Cluster"), "Audio Driver"=w329, "RecDeviceID"=w331) -> (w330:cluster{"RecDeviceID":u32, "Audio Driver":u32})
                    n158 = case shown="True" w356 {
                      tunnel: w358 -> [_ w431]
                      tunnel: [w399 w426] -> w357
                      tunnel: w353 -> [_ w422]
                      tunnel: w351 -> [_ w430]
                      tunnel: w350 -> [_ w429]
                      tunnel: w355 -> [w399 w428]
                      tunnel: w354 -> [_ w425]
                      tunnel: w331 -> [_ w421]
                      tunnel: w349 -> [_ w418]
                      tunnel: w348 -> [_ w419]
                      tunnel: w347 -> [_ w414]
                      tunnel: w346 -> [_ w424]
                      tunnel: w345 -> [_ w420]
                      tunnel: w344 -> [_ w423]
                      tunnel: w335 -> [_ w409]
                      tunnel: w341 -> [_ w413]
                      tunnel: w337 -> [_ w412]
                      tunnel: w336 -> [_ w411]
                      tunnel: w334 -> [_ w407]
                      tunnel: [w398 w401] -> w326
                      tunnel: w327 -> [w398 w400]
                      tunnel: w330 -> [_ w404]
                      tunnel: w329 -> [_ w403]
                      tunnel: w328 -> [_ _]
                      frame False {
                      }
                      frame True {
                        w410 = cluster{"X0":dbl, "dX":dbl, "Y":sgl[]} {"X0"=0.0, "dX"=0.0, "Y"=[]}  # Waveform
                        n159 = for {
                          tunnel: w422 -> [w454] mode=indexing
                          tunnel: [w453] -> w417 mode=indexing
                          tunnel: [w452] -> w416 mode=indexing
                          tunnel: [w451] -> w415 mode=indexing
                          tunnel: w420 -> [w450]
                          tunnel: w419 -> [w449]
                          tunnel: w418 -> [w448]
                          tunnel: w414 -> [w447]
                          tunnel: [w446] -> w405 mode=indexing
                          tunnel: w404 -> [w445]
                          n160 = local read "Index for testinfor"() -> (w443:i32)
                          n161 = call "CRYAcq Get Channel Name.vi"("I_channel Info Out"=w448, "O_channel Info Out"=w447, "Cluster"=w445, "RecChannel"=w454, "Selected Play In"=w449, "Index for testinfor"=w443, "Acquisition Type"=w450) -> ("Vmax In"=w446:dbl, "ChannelName In"=w453:string, "Test Info"=w452:string, "Latency (samples) In"=w451:dbl)  [unwired: 3 in, 2 out]
                          n162 = Increment(x=w443) -> (x+1=w444:i32)
                          n163 = local write "Index for testinfor"(w444) -> ()
                        }
                        n164 = Reciprocal(x=w409) -> (1/x=w408:dbl)
                        n165 = for {
                          tunnel: w431 -> [w499]
                          tunnel: [w498] -> w427 mode=indexing
                          tunnel: w422 -> [w468] mode=indexing
                          tunnel: w410 -> [w497]
                          tunnel: w430 -> [w494]
                          tunnel: w429 -> [w474]
                          tunnel: w408 -> [w489]
                          tunnel: w425 -> [w487]
                          tunnel: w421 -> [w485]
                          tunnel: w418 -> [w484]
                          tunnel: w424 -> [w480]
                          tunnel: w423 -> [w461]
                          tunnel: w409 -> [w464]
                          tunnel: w417 -> [w466] mode=indexing
                          tunnel: w416 -> [w473] mode=indexing
                          tunnel: w415 -> [w455] mode=indexing
                          tunnel: w413 -> [w470]
                          tunnel: w412 -> [w457] mode=indexing
                          tunnel: w411 -> [w463]
                          tunnel: w407 -> [w460]
                          tunnel: [w459] -> w406 mode=indexing
                          tunnel: w405 -> [_] mode=indexing
                          tunnel: [w457] -> w402 mode=indexing
                          tunnel: w403 -> [w456]
                          w479 = FALSE ("Overload?")
                          w490 = TRUE ("display Y")
                          w493 = u16 1  # lin
                          # "For recoding mode, delay non-consideration??"
                          n166 = call "CRYGet Channel Calc Factor.vi"("Signal Path"=w457, "Channel Name"=w466, "Audio Driver"=w456, "Is Input?"=TRUE, "I/O_channel Info"=w484, "Channel(LR)"=w468, "DeviceID"=w485) -> ("Y unit"=w478:string, "Calibration All Cluster"=w458:T9, "Calc Factor"=w469:dbl)  [unwired: 2 out]
                          n167 = Select(t=w455, s=w461, f=0.0) -> ()  [unwired: 1 out]
                          n168 = case shown="0, Default" w468 {
                            tunnel: [w503 w522] -> w488
                            tunnel: w474 -> [_ w529]
                            tunnel: w494 -> [w511 _]
                            tunnel: [w505 w523] -> w465
                            tunnel: w455 -> [w507 w525]
                            tunnel: w480 -> [w501 w519]
                            tunnel: w461 -> [w510 w528]
                            tunnel: w457 -> [w504 w521]
                            tunnel: w463 -> [w502 w520]
                            tunnel: w455 -> [w500 w518]
                            frame 0, Default {
                              n169 = Array Size(array=w511) -> (size(s)=w508:i32)
                              n170 = Subtract(x=w508, y=w507) -> (x-y=w506:dbl)
                              n171 = Select(t=w506, s=w510, f=w508) -> (s? t:f=w509:dbl)
                              n172 = Array Subset(array=w511, index=w500, length=w509) -> (w505:i32[])
                              n173 = case shown="True" w501 {
                                tunnel: [w512 w517] -> w503
                                tunnel: w504 -> [_ w516]
                                tunnel: w502 -> [w512 w513]
                                frame False {
                                }
                                frame True {
                                n174 = Concatenate Strings(w513, " [" ("string"), w516, "]" ("string")) -> (w517:string)
                                }
                              }
                            }
                            frame 1 {
                              n175 = Array Size(array=w529) -> (size(s)=w526:i32)
                              n176 = Subtract(x=w526, y=w525) -> (x-y=w524:dbl)
                              n177 = Select(t=w524, s=w528, f=w526) -> (s? t:f=w527:dbl)
                              n178 = Array Subset(array=w529, index=w518, length=w527) -> (w523:i32[])
                              n179 = case shown="True" w519 {
                                tunnel: [w530 w535] -> w522
                                tunnel: w521 -> [_ w534]
                                tunnel: w520 -> [w530 w531]
                                frame False {
                                }
                                frame True {
                                n180 = Concatenate Strings(w531, " [" ("string"), w534, "]" ("string")) -> (w535:string)
                                }
                              }
                            }
                          }
                          n181 = Multiply(x=w465, y=w469) -> (x*y=w467:dbl[])
                          n182 = Flatten To String(anything=w458) -> (data string=w471:string)  [unwired: 1 in, 4 out]
                          n183 = To Single Precision Float(number=w467) -> (single precision float=w475:sgl[])
                          n184 = Array Size(array=w467) -> (size(s)=w472:i32)
                          n185 = Bundle By Name(cluster=w497, "X0"=0.0, "dX"=w489, "Y"=w475) -> (w496:cluster{"X0":dbl, "dX":dbl, "Y":sgl[]})
                          n186 = call "CRYUnflatten Test Infor.vi"("Falattend test infor"=w473) -> ("unflattened test infor data"=w482:T19)  [unwired: 9 out]
                          n187 = Bundle By Name(cluster=w482, "Signal Type"=w457, "In/Out"=TRUE, "Sampling Rate"=w464, "Samples"=w472, "Calibration Param"=w471, "Anti Alias"=w470) -> (w481:T19)
                          n188 = call "CRYFlatten Test Infor.vi"("Test Infor data"=w481) -> ("Fattened Data"=w483:string)  [unwired: 10 out]
                          n189 = Bundle By Name(cluster=w499, "Name"=w488, "Waveform"=w496, "X data"=w493, "Y data"=w493, "Y axis"=w493, "X unit"="s", "Y unit"=w478, "Y dB ref"=1.0, "display Y"=w490, "display X"=w490, "Overload?"=w479, "protected"=w479, "Signal Channel ID"=w468, "Test Info"=w483, "Step No."=w487, "Plot Settings.Color"=u32 16770066) -> (w498:T3)
                          n190 = Search 1D Array(1D array=w460, element=w457) -> (index of element=w459:i32)  [unwired: 1 in]
                        }
                        n191 = disable-structure shown="Enabled" {
                          disable-tunnel: w428 -> [w434 w436]
                          disable-tunnel: w427 -> [w433 w437]
                          disable-tunnel: [w432 w435] -> w426
                          disable-tunnel: w406 -> [_ w438]
                          frame Disabled {
                            n192 = Insert Into Array(array=w434, new element=w433) -> (w432:T3[])  [unwired: 1 in]
                          }
                          frame Enabled {
                            n193 = for {
                              tunnel: w438 -> [w441] mode=indexing
                              tunnel: w437 -> [w440] mode=indexing
                              shift-right: [w439] -> w435
                              shift-left: w436 -> [w442]
                              n194 = Replace Array Subset(array=w442, new element=w440, index=w441) -> (w439:T3[])
                            }
                          }
                        }
                        n195 = Build Array (concatenate)(w400, w402) -> (w401:string[])
                      }
                    }
                  }
                  n196 = Array Size(array=w253) -> (size(s)=w256:i32)
                  n197 = Initialize Array(1.0 ("element"), w256) -> (w254:dbl[])
                  n198 = Initialize Array(w257, 0 ("Dimension Size")) -> ()  [unwired: 1 out]
                  n199 = call "CRYGet Max FSD In.vi"("Signal Path"=w249, "use ch name"=w252, "Wave in"=w253, "Max Level"=w254, "Step No."=w251) -> ("Data Out"=w248:T1[])  [unwired: 6 in]
                }
              }
            }
            frame 2 {
              n200 = flat-sequence {
                tunnel: w542 -> [w548]
                tunnel: w541 -> [w553]
                tunnel: w540 -> [w552]
                tunnel: w539 -> [w551]
                frame #0 {
                  n201 = Unbundle By Name(w548) -> ("sine gen setting"=w547:string)
                  n202 = call "CRYUnflatten Signal Generator.vi"("Flat Signal Gen'r settings"=w547) -> ("Signal Gen'r settings"=w546:T20)  [unwired: 10 out]
                  n203 = global write "CRYMisc vis settings global.vi" "Signal Gen'r settings"(w546) -> ()
                }
                frame #1 {
                  n204 = call "CRYSignal Generator.vi"("Manual"=FALSE, "Execution control"=w551, "Mute"=TRUE, "Hardware in"=w553, "Calibration in"=w552) -> ()  [unwired: 5 in, 6 out]
                }
              }
              n205 = Initialize Array(w544, 0 ("Dimension Size")) -> (w543:T1[])
              n206 = Initialize Array(w537, 0 ("Dimension Size")) -> (w536:T3[])
            }
            frame 3 {
              n207 = flat-sequence {
                tunnel: w560 -> [w569]
                tunnel: [w575] -> w564
                tunnel: [w574] -> w563
                tunnel: w562 -> [w571]
                tunnel: w561 -> [w572]
                tunnel: w559 -> [w570]
                frame #0 {
                  n208 = Unbundle By Name(w569) -> ("voltmeter setting"=w568:string)
                  n209 = call "CRYUnflatten Multimeter.vi"("Flat Voltmeter setup"=w568) -> ("Voltmeter Settings"=w567:T21)  [unwired: 10 out]
                  n210 = global write "CRYMisc vis settings global.vi" "Voltmeter Settings"(w567) -> ()
                }
                frame #1 {
                  n211 = call "CRYMultimeter.vi"("Calibration in"=w572, "Hardware in"=w571, "Manual"=FALSE, "Execution control"=w570) -> ("Canceled?"=w575:bool, "InputLevel Out"=w574:T22)  [unwired: 7 in, 7 out]
                }
              }
              n212 = case shown="False" w564 {
                tunnel: w566 -> [w591 w596]
                tunnel: w563 -> [w581 _]
                tunnel: [w585 w595] -> w565
                tunnel: w555 -> [w584 _]
                tunnel: w554 -> [w577 _]
                frame False {
                  w582 = FALSE ("Bundle Element")
                  w587 = 0.0 ("Bundle Element")
                  w583 = TRUE ("Bundle Element")
                  w592 = 1.0
                  w590 = ""
                  w593 = u16 1  # lin
                  w594 = u16 1  # lin
                  n213 = Unbundle By Name(w581) -> ("InputLevel"=w580:dbl, "unit"=w579:string, "dB ref."=w578:dbl)
                  n214 = Index Array(array=w577) -> (element=w576:string)  [unwired: 1 in]
                  n215 = Bundle("Bundle Element"=w587, "InputLevel"=w580, "Bundle Element"=w587) -> (w589:T23)  [unwired: 1 out]
                  n216 = Build Array(w589) -> (w588:T24)
                  n217 = Bundle By Name(cluster=w591, "Name"=w576, "Curve"=w588, "X data"=w594, "Y data"=w594, "Z data"=w594, "X axis"=w593, "Y axis"=w593, "Z axis"=w593, "X unit"=w590, "Y unit"=w579, "Z unit"=w590, "X dB ref"=w592, "Y dB ref"=w578, "Z dB ref"=w592, "single val"=w583, "Step No."=w584, "display X"=w582, "display Y"=w583, "display Z"=w582) -> (w586:T1)
                  n218 = Build Array(w586) -> (w585:T1[])
                }
                frame True {
                  n219 = Initialize Array(w596, 0 ("Dimension Size")) -> (w595:T1[])
                }
              }
              n220 = Initialize Array(w557, 0 ("Dimension Size")) -> (w556:T3[])
            }
            frame 4 {
              n221 = flat-sequence {
                tunnel: w609 -> [w650]
                tunnel: w611 -> [w658]
                tunnel: w610 -> [w657]
                tunnel: w608 -> [w654]
                tunnel: [w653] -> w605
                tunnel: [w652] -> w604
                tunnel: [w651] -> w602
                frame #0 {
                  n222 = Unbundle By Name(w650) -> ("scope_fft setting"=w649:string)
                  n223 = call "CRYUnflatten Scope-FFT.vi"("Flat Scope-FFT setup"=w649) -> ("Scope-FFT settings"=w648:T25)  [unwired: 10 out]
                  n224 = global write "CRYMisc vis settings global.vi" "Scope-FFT settings"(w648) -> ()
                }
                frame #1 {
                  w655 = u32 0 items=["Time", "Spectrum"] ("Mode")
                  n225 = call "CRYScope-FFT.vi"("Mode"=w655, "Hardware"=w658, "Execution control"=w654, "Manual"=FALSE, "Calibration"=w657) -> ("Data cluster"=w652:T26, "Selected Signal Path"=w651:string, "Canceled"=w653:bool)  [unwired: 7 in, 5 out]
                }
              }
              n226 = case shown="False" w605 {
                tunnel: w607 -> [w641 w646]
                tunnel: [w613 w645] -> w606
                tunnel: w604 -> [w630 _]
                tunnel: w603 -> [w617 _]
                tunnel: w602 -> [w612 _]
                tunnel: w601 -> [w623 _]
                tunnel: w600 -> [_ w643]
                tunnel: [w618 w642] -> w599
                tunnel: w598 -> [w614 _]
                frame False {
                  w631 = u16 1 ("Y data")
                  w639 = TRUE ("display X")
                  n227 = Unbundle By Name(w630) -> ("Fs"=w628:dbl, "Y"=w629:dbl[], "Y Unit"=w627:string, "db ref"=w626:dbl)  [unwired: 1 out]
                  n228 = call "CRYGet Current Calibration Info.vi"("Is Input?"=TRUE, "Signal Type Name"=w612) -> ("Calibration All Cluster"=w622:T9)  [unwired: 9 out]
                  n229 = Index Array(array=w623) -> (element=w615:string)  [unwired: 1 in]
                  n230 = Flatten To String(anything=w622) -> (data string=w625:string)  [unwired: 1 in, 4 out]
                  n231 = Reciprocal(x=w628) -> (1/x=w633:dbl)
                  n232 = call "CRYUnflatten Test Infor.vi"() -> ("unflattened test infor data"=w638:T19)  [unwired: 1 in, 9 out]
                  n233 = Bundle By Name(cluster=w638, "Stimulus Type"="Frequency Stepped Sweep", "Signal Type"=w612, "In/Out"=TRUE, "Sampling Rate"=w628, "Calibration Param"=w625) -> (w637:T19)
                  n234 = call "CRYFlatten Test Infor.vi"("Test Infor data"=w637) -> ("Fattened Data"=w635:string)  [unwired: 10 out]
                  n235 = Bundle By Name(cluster=w641, "Name"=w615, "Waveform.dX"=w633, "Waveform.Y"=w629, "Step No."=w617, "X data"=w631, "Y data"=w631, "X unit"="s", "Y unit"=w627, "Y dB ref"=w626, "display X"=w639, "display Y"=w639, "Test Info"=w635) -> (w640:T3)
                  n236 = Build Array(w640) -> (w613:T3[])
                  n237 = Build Array(w612) -> (w616:string[])
                  n238 = Array Size(array=w613) -> (size(s)=w619:i32)
                  n239 = Initialize Array(1.0 ("element"), w619) -> (w621:dbl[])
                  n240 = call "CRYGet Max FSD In.vi"("Signal Path"=w616, "use ch name"=w614, "Wave in"=w613, "Max Level"=w621, "Step No."=w617) -> ("Data Out"=w618:T1[])  [unwired: 6 in]
                }
                frame True {
                  n241 = Initialize Array(w646, 0 ("Dimension Size")) -> (w645:T3[])
                  n242 = Initialize Array(w643, 0 ("Dimension Size")) -> (w642:T1[])
                }
              }
            }
            frame 5 {
              n243 = flat-sequence {
                tunnel: w667 -> [w672]
                tunnel: w671 -> [w681]
                tunnel: w670 -> [w680]
                tunnel: [w678] -> w668
                tunnel: w666 -> [w676]
                tunnel: [w675] -> w662
                frame #0 {
                  n244 = Unbundle By Name(w672) -> ("scope_fft setting"=w674:string)
                  n245 = call "CRYUnflatten Scope-FFT.vi"("Flat Scope-FFT setup"=w674) -> ("Scope-FFT settings"=w673:T25)  [unwired: 10 out]
                  n246 = global write "CRYMisc vis settings global.vi" "Scope-FFT settings"(w673) -> ()
                }
                frame #1 {
                  w679 = u32 1 items=["Time", "Spectrum"] ("Mode")
                  n247 = call "CRYScope-FFT.vi"("Mode"=w679, "Hardware"=w681, "Execution control"=w676, "Manual"=FALSE, "Calibration"=w680) -> ("Data cluster"=w675:T26, "Canceled"=w678:bool)  [unwired: 7 in, 6 out]
                }
              }
              n248 = case "canceled?" shown="False" w668 {
                tunnel: [w697 w715] -> w669
                tunnel: w662 -> [w691 _]
                tunnel: w661 -> [w695 _]
                tunnel: w660 -> [w694 w714]
                tunnel: w659 -> [w683 _]
                frame False {
                  w692 = TRUE ("Bundle Element")
                  w693 = FALSE ("Bundle Element")
                  w700 = 1.0
                  w701 = u16 1  # lin
                  w702 = u16 1  # lin
                  n249 = Unbundle By Name(w691) -> ("df"=w684:dbl, "Y"=w690:dbl[], "Y axis"=w686:u16, "Y Unit"=w689:string, "db ref"=w685:dbl)
                  n250 = for {
                    tunnel: w684 -> [w713]
                    tunnel: w690 -> [w711] mode=indexing
                    tunnel: [w708] -> w696 mode=indexing
                    i -> [w712]
                    n251 = Multiply(x=w713, y=w712) -> (x*y=w709:dbl)
                    n252 = Bundle(w709, w711, 0.0) -> (w708:cluster{dbl, dbl, dbl})  [unwired: 1 out]
                  }
                  n253 = case shown="0, Default" w686 {
                    tunnel: w689 -> [w705 w707]
                    tunnel: w685 -> [w704 _]
                    tunnel: [w703 w707] -> w688
                    frame 0, Default {
                      n254 = Format Into String(format string="dB re %.p %s", w704, w705) -> (resulting string=w703:string)  [unwired: 2 in, 1 out]
                    }
                    frame 1 {
                    }
                  }
                  n255 = Index Array(array=w683) -> (element=w682:string)  [unwired: 1 in]
                  n256 = Bundle By Name(cluster=w694, "Name"=w682, "Curve"=w696, "X data"=w702, "Y data"=w686, "Z data"=w702, "X axis"=w701, "Y axis"=w701, "Z axis"=w701, "X unit"="Hz", "Y unit"=w688, "Z unit"="", "X dB ref"=w700, "Y dB ref"=w685, "Z dB ref"=w700, "single val"=w693, "Step No."=w695, "display X"=w692, "display Y"=w692, "display Z"=w693) -> (w698:T1)
                  n257 = Build Array(w698) -> (w697:T1[])
                }
                frame True {
                  n258 = Initialize Array(w714, 0 ("Dimension Size")) -> (w715:T1[])
                }
              }
              n259 = Initialize Array(w664, 0 ("Dimension Size")) -> (w663:T3[])
            }
            frame 6 {
              n260 = flat-sequence {
                tunnel: w726 -> [w732]
                tunnel: w731 -> [w743]
                tunnel: w730 -> [w742]
                tunnel: [w740] -> w728
                tunnel: [w739] -> _
                tunnel: w725 -> [w738]
                tunnel: [w737] -> w720
                tunnel: [w736] -> w719
                tunnel: [w735] -> w717
                frame #0 {
                  n261 = Unbundle By Name(w732) -> ("rta setting"=w733:string)
                  n262 = call "CRYUnflatten RTA.vi"("Flat RTA setup"=w733) -> ("RTA settings"=w734:T27)  [unwired: 10 out]
                  n263 = global write "CRYMisc vis settings global.vi" "RTA settings"(w734) -> ()
                }
                frame #1 {
                  n264 = call "CRYRTA.vi"("Manual"=FALSE, "Hardware in"=w743, "Execution control"=w738, "Calibration in"=w742) -> ("Canceled?"=w740:bool, "band power"=w737:dbl[], "Data output"=w735:T28, "df Array"=w736:dbl[], "Data Out"=w739:T1)  [unwired: 5 in, 2 out]
                }
              }
              n265 = case "canceled?" shown="False" w728 {
                tunnel: [w760 w772] -> w727
                tunnel: w729 -> [w759 w773]
                tunnel: w717 -> [w751 _]
                tunnel: w721 -> [w745 _]
                tunnel: w720 -> [w758 _]
                tunnel: w719 -> [w757 _]
                tunnel: w718 -> [w756 _]
                frame False {
                  w752 = u16 0  # db
                  w754 = TRUE ("Bundle Element")
                  w764 = 1.0
                  w746 = u16 1  # lin
                  w765 = u16 1  # lin
                  n266 = Unbundle By Name(w751) -> ("db ref"=w747:dbl, "Y Unit"=w748:string)
                  n267 = for {
                    tunnel: w757 -> [w771] mode=indexing
                    tunnel: w758 -> [w769] mode=indexing
                    tunnel: [w766] -> w761 mode=indexing
                    i -> [w770]
                    n268 = Multiply(x=w771, y=w770) -> (x*y=w767:dbl)
                    n269 = Bundle(w767, w769, 0.0) -> (w766:cluster{dbl, dbl, dbl})  [unwired: 1 out]
                  }
                  n270 = Format Into String(format string="dB re %.p %s", w747, w748) -> (resulting string=w749:string)  [unwired: 2 in, 1 out]
                  n271 = Index Array(array=w745) -> (element=w744:string)  [unwired: 1 in]
                  n272 = Bundle By Name(cluster=w759, "Name"=w744, "Curve"=w761, "X data"=w765, "Y data"=w752, "Z data"=w765, "X axis"=w746, "Y axis"=w746, "Z axis"=w746, "X unit"="Hz", "Y unit"=w749, "Z unit"="", "X dB ref"=w764, "Y dB ref"=w747, "Z dB ref"=w764, "single val"=FALSE ("Bundle Element"), "Step No."=w756, "display X"=w754, "display Y"=w754, "display Z"=w754) -> (w762:T1)
                  n273 = Build Array(w762) -> (w760:T1[])
                }
                frame True {
                  n274 = Initialize Array(w773, 0 ("Dimension Size")) -> (w772:T1[])
                }
              }
              n275 = Initialize Array(w723, 0 ("Dimension Size")) -> (w722:T3[])
            }
            frame 7 {
              n276 = flat-sequence {
                tunnel: w782 -> [w791]
                tunnel: [w801] -> w786
                tunnel: [w800] -> w785
                tunnel: w784 -> [w794]
                tunnel: w783 -> [w795]
                tunnel: w781 -> [w799]
                tunnel: w780 -> [w796]
                frame #0 {
                  n277 = Unbundle By Name(w791) -> ("sine gen setting"=w793:string, "voltmeter setting"=w790:string)
                  n278 = call "CRYUnflatten Signal Generator.vi"("Flat Signal Gen'r settings"=w793) -> ("Signal Gen'r settings"=w792:T20)  [unwired: 10 out]
                  n279 = call "CRYUnflatten Multimeter.vi"("Flat Voltmeter setup"=w790) -> ("Voltmeter Settings"=w789:T21)  [unwired: 10 out]
                  n280 = global write "CRYMisc vis settings global.vi" "Signal Gen'r settings"(w792) -> ()
                  n281 = global write "CRYMisc vis settings global.vi" "Voltmeter Settings"(w789) -> ()
                }
                frame #1 {
                  w802 = FALSE ("Manual")
                  n282 = stacked-sequence {
                    tunnel: w799 -> [w804]
                    tunnel: [w803] -> w798
                    frame #0 {
                      n283 = Wait (ms)(milliseconds to wait=w804) -> ()  [unwired: 1 out]
                      n284 = local read "Record [ms]"() -> (w803:dbl)
                    }
                  }
                  n285 = call "CRYSignal Generator.vi"("Manual"=w802, "Execution control"=w796, "Mute"=TRUE, "Hardware in"=w795, "Calibration in"=w794) -> ()  [unwired: 5 in, 6 out]
                  n286 = call "CRYMultimeter.vi"("Time(sec)"=w798, "Calibration in"=w794, "Hardware in"=w795, "Manual"=w802, "Execution control"=w796) -> ("Canceled?"=w801:bool, "InputLevel Out"=w800:T22)  [unwired: 6 in, 7 out]
                }
              }
              n287 = case shown="False" w786 {
                tunnel: w787 -> [w820 w825]
                tunnel: w785 -> [w810 _]
                tunnel: [w814 w824] -> w788
                tunnel: w776 -> [w806 _]
                tunnel: w775 -> [w813 _]
                frame False {
                  w811 = FALSE ("display X")
                  w816 = 0.0 ("Bundle Element")
                  w812 = TRUE ("Bundle Element")
                  w821 = 1.0
                  w819 = ""
                  w822 = u16 1  # lin
                  w823 = u16 1  # lin
                  n288 = Unbundle By Name(w810) -> ("InputLevel"=w809:dbl, "unit"=w808:string, "dB ref."=w807:dbl)
                  n289 = Index Array(array=w806) -> (element=w805:string)  [unwired: 1 in]
                  n290 = Bundle("Bundle Element"=w816, "InputLevel"=w809, "Bundle Element"=w816) -> (w818:T23)  [unwired: 1 out]
                  n291 = Build Array(w818) -> (w817:T24)
                  n292 = Bundle By Name(cluster=w820, "Name"=w805, "Curve"=w817, "X data"=w823, "Y data"=w823, "Z data"=w823, "X axis"=w822, "Y axis"=w822, "Z axis"=w822, "X unit"=w819, "Y unit"=w808, "Z unit"=w819, "X dB ref"=w821, "Y dB ref"=w807, "Z dB ref"=w821, "single val"=w812, "Step No."=w813, "display X"=w811, "display Y"=w812, "display Z"=w811) -> (w815:T1)
                  n293 = Build Array(w815) -> (w814:T1[])
                }
                frame True {
                  n294 = Initialize Array(w825, 0 ("Dimension Size")) -> (w824:T1[])
                }
              }
              n295 = Initialize Array(w778, 0 ("Dimension Size")) -> (w777:T3[])
            }
            frame 8 {
              n296 = flat-sequence {
                tunnel: w839 -> [w880]
                tunnel: w841 -> [w893]
                tunnel: w840 -> [w892]
                tunnel: w838 -> [w889]
                tunnel: w837 -> [w886]
                tunnel: [w885] -> w836
                tunnel: [w884] -> w832
                tunnel: [w883] -> w830
                frame #0 {
                  n297 = Unbundle By Name(w880) -> ("sine gen setting"=w882:string, "scope_fft setting"=w878:string)
                  n298 = call "CRYUnflatten Signal Generator.vi"("Flat Signal Gen'r settings"=w882) -> ("Signal Gen'r settings"=w881:T20)  [unwired: 10 out]
                  n299 = call "CRYUnflatten Scope-FFT.vi"("Flat Scope-FFT setup"=w878) -> ("Scope-FFT settings"=w879:T25)  [unwired: 10 out]
                  n300 = global write "CRYMisc vis settings global.vi" "Signal Gen'r settings"(w881) -> ()
                  n301 = global write "CRYMisc vis settings global.vi" "Scope-FFT settings"(w879) -> ()
                }
                frame #1 {
                  w890 = FALSE ("Manual")
                  w891 = u32 0 items=["Time", "Spectrum"] ("Mode")
                  n302 = stacked-sequence {
                    tunnel: w889 -> [w895]
                    tunnel: [w894] -> w888
                    frame #0 {
                      n303 = Wait (ms)(milliseconds to wait=w895) -> ()  [unwired: 1 out]
                      n304 = local read "Record [ms]"() -> (w894:dbl)
                    }
                  }
                  n305 = call "CRYSignal Generator.vi"("Manual"=w890, "Execution control"=w886, "Mute"=TRUE, "Hardware in"=w893, "Calibration in"=w892) -> ()  [unwired: 5 in, 6 out]
                  n306 = call "CRYScope-FFT.vi"("Mode"=w891, "Time(sec)"=w888, "Hardware"=w893, "Execution control"=w886, "Manual"=w890, "Calibration"=w892) -> ("Data cluster"=w884:T26, "Selected Signal Path"=w883:string, "Canceled"=w885:bool)  [unwired: 6 in, 5 out]
                }
              }
              n307 = case shown="False" w836 {
                tunnel: w835 -> [w871 w876]
                tunnel: [w846 w875] -> w834
                tunnel: w833 -> [w853 _]
                tunnel: w832 -> [w862 _]
                tunnel: w831 -> [w845 _]
                tunnel: w830 -> [w847 _]
                tunnel: w829 -> [w844 _]
                tunnel: w828 -> [_ w873]
                tunnel: [w843 w872] -> w827
                frame False {
                  w857 = u16 1 ("X data")
                  w869 = TRUE ("display X")
                  n308 = Unbundle By Name(w862) -> ("Fs"=w861:dbl, "Y"=w842:dbl[], "db ref"=w860:dbl, "Y Unit"=w858:string)  [unwired: 1 out]
                  n309 = Index Array(array=w853) -> (element=w852:string)  [unwired: 1 in]
                  n310 = call "CRYGet Current Calibration Info.vi"("Is Input?"=TRUE, "Signal Type Name"=w847) -> ("Calibration All Cluster"=w854:T9)  [unwired: 9 out]
                  n311 = Flatten To String(anything=w854) -> (data string=w856:string)  [unwired: 1 in, 4 out]
                  n312 = call "CRYUnflatten Test Infor.vi"() -> ("unflattened test infor data"=w868:T19)  [unwired: 1 in, 9 out]
                  n313 = Bundle By Name(cluster=w868, "Stimulus Type"="Frequency Stepped Sweep", "Signal Type"=w847, "In/Out"=TRUE, "Sampling Rate"=w861, "Calibration Param"=w856) -> (w867:T19)
                  n314 = Reciprocal(x=w861) -> (1/x=w863:dbl)
                  n315 = call "CRYFlatten Test Infor.vi"("Test Infor data"=w867) -> ("Fattened Data"=w864:string)  [unwired: 10 out]
                  n316 = Bundle By Name(cluster=w871, "Name"=w852, "Waveform.dX"=w863, "Waveform.Y"=w842, "Step No."=w845, "X data"=w857, "Y data"=w857, "Y dB ref"=w860, "X unit"="s", "Y unit"=w858, "display X"=w869, "display Y"=w869, "Test Info"=w864) -> (w870:T3)
                  n317 = Build Array(w870) -> (w846:T3[])
                  n318 = Build Array(w847) -> (w848:string[])
                  n319 = Array Size(array=w846) -> (size(s)=w849:i32)
                  n320 = Initialize Array(1.0 ("element"), w849) -> (w851:dbl[])
                  n321 = call "CRYGet Max FSD In.vi"("Signal Path"=w848, "use ch name"=w844, "Wave in"=w846, "Max Level"=w851, "Step No."=w845) -> ("Data Out"=w843:T1[])  [unwired: 6 in]
                }
                frame True {
                  n322 = Initialize Array(w876, 0 ("Dimension Size")) -> (w875:T3[])
                  n323 = Initialize Array(w873, 0 ("Dimension Size")) -> (w872:T1[])
                }
              }
            }
            frame 9 {
              n324 = flat-sequence {
                tunnel: w903 -> [w910]
                tunnel: w909 -> [w924]
                tunnel: w908 -> [w923]
                tunnel: [w921] -> w907
                tunnel: w904 -> [w920]
                tunnel: w902 -> [w916]
                tunnel: [w915] -> w897
                frame #0 {
                  n325 = Unbundle By Name(w910) -> ("sine gen setting"=w914:string, "scope_fft setting"=w911:string)
                  n326 = call "CRYUnflatten Signal Generator.vi"("Flat Signal Gen'r settings"=w914) -> ("Signal Gen'r settings"=w913:T20)  [unwired: 10 out]
                  n327 = call "CRYUnflatten Scope-FFT.vi"("Flat Scope-FFT setup"=w911) -> ("Scope-FFT settings"=w912:T25)  [unwired: 10 out]
                  n328 = global write "CRYMisc vis settings global.vi" "Signal Gen'r settings"(w913) -> ()
                  n329 = global write "CRYMisc vis settings global.vi" "Scope-FFT settings"(w912) -> ()
                }
                frame #1 {
                  w918 = FALSE ("Manual")
                  w922 = u32 1 items=["Time", "Spectrum"] ("Mode")
                  n330 = stacked-sequence {
                    tunnel: w920 -> [w926]
                    tunnel: [w925] -> w919
                    frame #0 {
                      n331 = Wait (ms)(milliseconds to wait=w926) -> ()  [unwired: 1 out]
                      n332 = local read "Record [ms]"() -> (w925:dbl)
                    }
                  }
                  n333 = call "CRYSignal Generator.vi"("Manual"=w918, "Execution control"=w916, "Mute"=TRUE, "Hardware in"=w924, "Calibration in"=w923) -> ()  [unwired: 5 in, 6 out]
                  n334 = call "CRYScope-FFT.vi"("Mode"=w922, "Time(sec)"=w919, "Hardware"=w924, "Execution control"=w916, "Manual"=w918, "Calibration"=w923) -> ("Data cluster"=w915:T26, "Canceled"=w921:bool)  [unwired: 6 in, 6 out]
                }
              }
              n335 = case "canceled?" shown="False" w907 {
                tunnel: [w940 w959] -> w905
                tunnel: w906 -> [w941 w960]
                tunnel: w898 -> [w928 _]
                tunnel: w897 -> [w935 _]
                tunnel: w896 -> [w939 _]
                frame False {
                  w937 = TRUE ("Bundle Element")
                  w938 = FALSE ("Bundle Element")
                  w945 = 1.0
                  w946 = u16 1  # lin
                  w947 = u16 1  # lin
                  n336 = Unbundle By Name(w935) -> ("df"=w929:dbl, "Y"=w934:dbl[], "Y axis"=w932:u16, "Y Unit"=w936:string, "db ref"=w930:dbl)
                  n337 = Index Array(array=w928) -> (element=w927:string)  [unwired: 1 in]
                  n338 = for {
                    tunnel: w929 -> [w958]
                    tunnel: w934 -> [w956] mode=indexing
                    tunnel: [w953] -> w942 mode=indexing
                    i -> [w957]
                    n339 = Multiply(x=w958, y=w957) -> (x*y=w954:dbl)
                    n340 = Bundle(w954, w956, 0.0) -> (w953:cluster{dbl, dbl, dbl})  [unwired: 1 out]
                  }
                  n341 = case shown="0, Default" w932 {
                    tunnel: w936 -> [w950 w952]
                    tunnel: w930 -> [w949 _]
                    tunnel: [w948 w952] -> w933
                    frame 0, Default {
                      n342 = Format Into String(format string="dB re %.p %s", w949, w950) -> (resulting string=w948:string)  [unwired: 2 in, 1 out]
                    }
                    frame 1 {
                    }
                  }
                  n343 = Bundle By Name(cluster=w941, "Name"=w927, "Curve"=w942, "X data"=w947, "Y data"=w932, "Z data"=w947, "X axis"=w946, "Y axis"=w946, "Z axis"=w946, "X unit"="Hz", "Y unit"=w933, "Z unit"="", "X dB ref"=w945, "Y dB ref"=w930, "Z dB ref"=w945, "single val"=w938, "Step No."=w939, "display X"=w937, "display Y"=w937, "display Z"=w938) -> (w943:T1)
                  n344 = Build Array(w943) -> (w940:T1[])
                }
                frame True {
                  n345 = Initialize Array(w960, 0 ("Dimension Size")) -> (w959:T1[])
                }
              }
              n346 = Initialize Array(w900, 0 ("Dimension Size")) -> (w899:T3[])
            }
            frame 10 {
              n347 = flat-sequence {
                tunnel: w971 -> [w980]
                tunnel: w977 -> [w993]
                tunnel: [w992] -> w974
                tunnel: w973 -> [w990]
                tunnel: w972 -> [w988]
                tunnel: w970 -> [w986]
                tunnel: [w985] -> w965
                tunnel: [w984] -> w964
                tunnel: [w983] -> w962
                frame #0 {
                  n348 = Unbundle By Name(w980) -> ("sine gen setting"=w982:string, "rta setting"=w978:string)
                  n349 = call "CRYUnflatten Signal Generator.vi"("Flat Signal Gen'r settings"=w982) -> ("Signal Gen'r settings"=w981:T20)  [unwired: 10 out]
                  n350 = call "CRYUnflatten RTA.vi"("Flat RTA setup"=w978) -> ("RTA settings"=w979:T27)  [unwired: 10 out]
                  n351 = global write "CRYMisc vis settings global.vi" "Signal Gen'r settings"(w981) -> ()
                  n352 = global write "CRYMisc vis settings global.vi" "RTA settings"(w979) -> ()
                }
                frame #1 {
                  w991 = FALSE ("Manual")
                  n353 = stacked-sequence {
                    tunnel: w990 -> [w995]
                    tunnel: [w994] -> w989
                    frame #0 {
                      n354 = Wait (ms)(milliseconds to wait=w995) -> ()  [unwired: 1 out]
                      n355 = local read "Record [ms]"() -> (w994:dbl)
                    }
                  }
                  n356 = call "CRYSignal Generator.vi"("Manual"=w991, "Execution control"=w986, "Mute"=TRUE, "Hardware in"=w988, "Calibration in"=w993) -> ()  [unwired: 5 in, 6 out]
                  n357 = call "CRYRTA.vi"("Manual"=w991, "Avg. Time(sec)"=w989, "Hardware in"=w988, "Execution control"=w986, "Calibration in"=w993) -> ("Canceled?"=w992:bool, "band power"=w985:dbl[], "Data output"=w983:T28, "df Array"=w984:dbl[])  [unwired: 4 in, 3 out]
                }
              }
              n358 = case "canceled?" shown="False" w974 {
                tunnel: [w1009 w1025] -> w976
                tunnel: w975 -> [w1010 w1024]
                tunnel: w966 -> [w997 _]
                tunnel: w965 -> [w1008 _]
                tunnel: w964 -> [w1007 _]
                tunnel: w963 -> [w1006 _]
                tunnel: w962 -> [w1002 _]
                frame False {
                  w998 = u16 0  # db
                  w1005 = TRUE ("Bundle Element")
                  w1015 = 1.0
                  w1016 = u16 1  # lin
                  w1017 = u16 1  # lin
                  n359 = Unbundle By Name(w1002) -> ("db ref"=w1000:dbl, "Y Unit"=w1003:string)
                  n360 = Index Array(array=w997) -> (element=w996:string)  [unwired: 1 in]
                  n361 = Format Into String(format string="dB re %.p %s", w1000, w1003) -> (resulting string=w1001:string)  [unwired: 2 in, 1 out]
                  n362 = for {
                    tunnel: w1007 -> [w1023] mode=indexing
                    tunnel: w1008 -> [w1021] mode=indexing
                    tunnel: [w1018] -> w1011 mode=indexing
                    i -> [w1022]
                    n363 = Multiply(x=w1023, y=w1022) -> (x*y=w1019:dbl)
                    n364 = Bundle(w1019, w1021, 0.0) -> (w1018:cluster{dbl, dbl, dbl})  [unwired: 1 out]
                  }
                  n365 = Bundle By Name(cluster=w1010, "Name"=w996, "Curve"=w1011, "X data"=w1017, "Y data"=w998, "Z data"=w1017, "X axis"=w1016, "Y axis"=w1016, "Z axis"=w1016, "X unit"="Hz", "Y unit"=w1001, "Z unit"="", "X dB ref"=w1015, "Y dB ref"=w1000, "Z dB ref"=w1015, "single val"=FALSE ("Bundle Element"), "Step No."=w1006, "display X"=w1005, "display Y"=w1005, "display Z"=w1005) -> (w1012:T1)
                  n366 = Build Array(w1012) -> (w1009:T1[])
                }
                frame True {
                  n367 = Initialize Array(w1024, 0 ("Dimension Size")) -> (w1025:T1[])
                }
              }
              n368 = Initialize Array(w968, 0 ("Dimension Size")) -> (w967:T3[])
            }
            frame 11, Default {
              w1029 = ""
              w1030 = 44100.0 ("Fs")
              w1037 = u16 1 ("Y data")
              w1045 = TRUE ("display X")
              # "?????"
              # "??????"
              n369 = call "CRYGet Current Calibration Info.vi"("Is Input?"=TRUE, "Signal Type Name"=w1029) -> ("Calibration All Cluster"=w1034:T9)  [unwired: 9 out]
              n370 = Flatten To String(anything=w1034) -> (data string=w1036:string)  [unwired: 1 in, 4 out]
              n371 = Reciprocal(x=w1030) -> (1/x=w1039:dbl)
              n372 = call "CRYUnflatten Test Infor.vi"() -> ("unflattened test infor data"=w1044:T19)  [unwired: 1 in, 9 out]
              n373 = Bundle By Name(cluster=w1044, "Stimulus Type"="DC", "Signal Type"=w1029, "In/Out"=TRUE, "Sampling Rate"=w1030, "Calibration Param"=w1036) -> (w1043:T19)
              n374 = Index Array(array=w1028) -> (element=w1027:string)  [unwired: 1 in]
              n375 = call "CRYFlatten Test Infor.vi"("Test Infor data"=w1043) -> ("Fattened Data"=w1041:string)  [unwired: 10 out]
              n376 = Bundle By Name(cluster=w1052, "Name"=w1027, "Waveform.dX"=w1039, "Waveform.Y"=sgl[] [], "Step No."=w1047, "X data"=w1037, "Y data"=w1037, "X unit"="s", "Y unit"="V", "Y dB ref"=1.0, "display X"=w1045, "display Y"=w1045, "Test Info"=w1041) -> (w1046:T3)
              n377 = Build Array(w1046) -> (w1051:T3[])
              n378 = Initialize Array(w1048, 0 ("Dimension Size")) -> (w1049:T1[])
            }
          }
          "Data out" <- w71
          "Wave out" <- w70
        }
        frame #2 {
          w1058 = 2.0 ("x")
          n379 = local read "Wave out"() -> (w1053:T3[])
          n380 = local read "Data out"() -> (w1063:T1[])
          n381 = Array Size(array=w1053) -> (size(s)=w1060:i32)
          n382 = Square Root(x=w1058) -> (sqrt(x)=w1059:dbl)
          n383 = Multiply(x=w1058, y=w1059) -> (x*y=w1057:dbl)
          n384 = Initialize Array(w1057, w1060) -> (w1056:dbl[])
          n385 = local read "Acquisition Type"() -> (w1069:u16)
          n386 = call "CRYGet Max FSD In.vi"("Wave in"=w1053, "Max Level"=w1056, "Step No."=w1061) -> ("Data Out"=w1062:T1[])  [unwired: 8 in]
          n387 = Build Array (concatenate)(w1063, w1062) -> (w1054:T1[])
          n388 = call "CRYAcq Save to Curve.vi"("Acquisition Type"=w1069, "Setup in"=w1065, "Data In"=w1054, "Wave In"=w1053, "Is Save?"=TRUE) -> ("Inserted Names Out"=→"Inserted Names Out":string[])  [unwired: 2 in, 8 out]
          n389 = call "CRYGet Type from Data.vi"("Waves"=w1053, "Values"=w1054) -> ("Type"=→"Types Out":string[])  [unwired: 9 in]
          n390 = local read "Verdict"() -> (w1066:bool)
          n391 = call "CRYUnflatten Results.vi"() -> ("Result"=w1067:T5)  [unwired: 1 in, 10 out]
          n392 = Bundle By Name(cluster=w1067, "Verdict"=w1066) -> (w1071:T5)
          n393 = Build Array(w1071) -> (→"Results out":T5[])
        }
      }
    }
  }
